vi "主界面.vi"() -> ()   [LabVIEW 2016]
uses:
  <vilib>/Utility/miscctls.llb/LVPointTypeDef.ctl
  <vilib>/NI/Modbus Library/API/Wrapper/Create Serial Slave.vi
  <vilib>/NI/Modbus Library/API/Slave/Modbus Slave.lvclass
  <vilib>/ptbypt/NI_PtbyPt.lvlib
  <vilib>/NI/Modbus Library/API/Wrapper/API Main.lvlib
panel:
  in  "质控单元串口重开":enum16{"不重开", "串口重开"}(ring)
  in  "采配水串口重开":enum16{"不重开", "串口重开"}(ring)
  out "质控运行中":bool
  out "质控单元通讯":bool
  out "采配水运行中":bool
  out "采配水通讯":bool
  out "CODCr运行中":bool
  out "CODMn运行中":bool
  out "总磷运行中":bool
  out "总氮运行中":bool
  out "氨氮运行中":bool
  out "CODCr通讯":bool
  out "CODMn通讯":bool
  out "总磷通讯":bool
  out "总氮通讯":bool
  out "氨氮通讯":bool
  out "系统日期/时间字符串":string
  in  "质控单元串口参数":T1={"VISA resource name"="COM28", "baud rate (设置)"=115200, "unit ID"=1}
  in  "采配水串口参数":T1={"VISA resource name"="COM23", "baud rate (设置)"=115200, "unit ID"=10}
  in  "质控单元":bool
  in  "采配水":bool
  in  "总磷串口参数":T1={"VISA resource name"="COM25", "baud rate (设置)"=115200, "unit ID"=1}
  in  "CODCr串口参数":T1={"VISA resource name"="COM29", "baud rate (设置)"=9600, "unit ID"=1}
  in  "CODMn串口参数":T1={"VISA resource name"="COM24", "baud rate (设置)"=115200, "unit ID"=1}
  in  "总氮串口参数":T1={"VISA resource name"="COM30", "baud rate (设置)"=115200, "unit ID"=2}
  in  "氨氮串口参数":T1={"VISA resource name"="COM27", "baud rate (设置)"=115200, "unit ID"=3}
  in  "CODCr":bool
  in  "CODMn":bool
  in  "总磷":bool
  in  "总氮":bool
  in  "氨氮":bool
  in  "CODCr串口重开":enum16{"不重开", "串口重开"}(ring)
  in  "CODMn串口重开":enum16{"不重开", "串口重开"}(ring)
  in  "总磷串口重开":enum16{"不重开", "串口重开"}(ring)
  in  "总氮串口重开":enum16{"不重开", "串口重开"}(ring)
  in  "氨氮串口重开":enum16{"不重开", "串口重开"}(ring)
  in  "退出":bool
  # "系统状态区"
  # "采配水"
  # "氨氮"
  # "总氮"
  # "总磷"
  # "CODMn"
  # "CODCr"
  # "质控单元"
  # "通讯状态："
  # "测量状态："
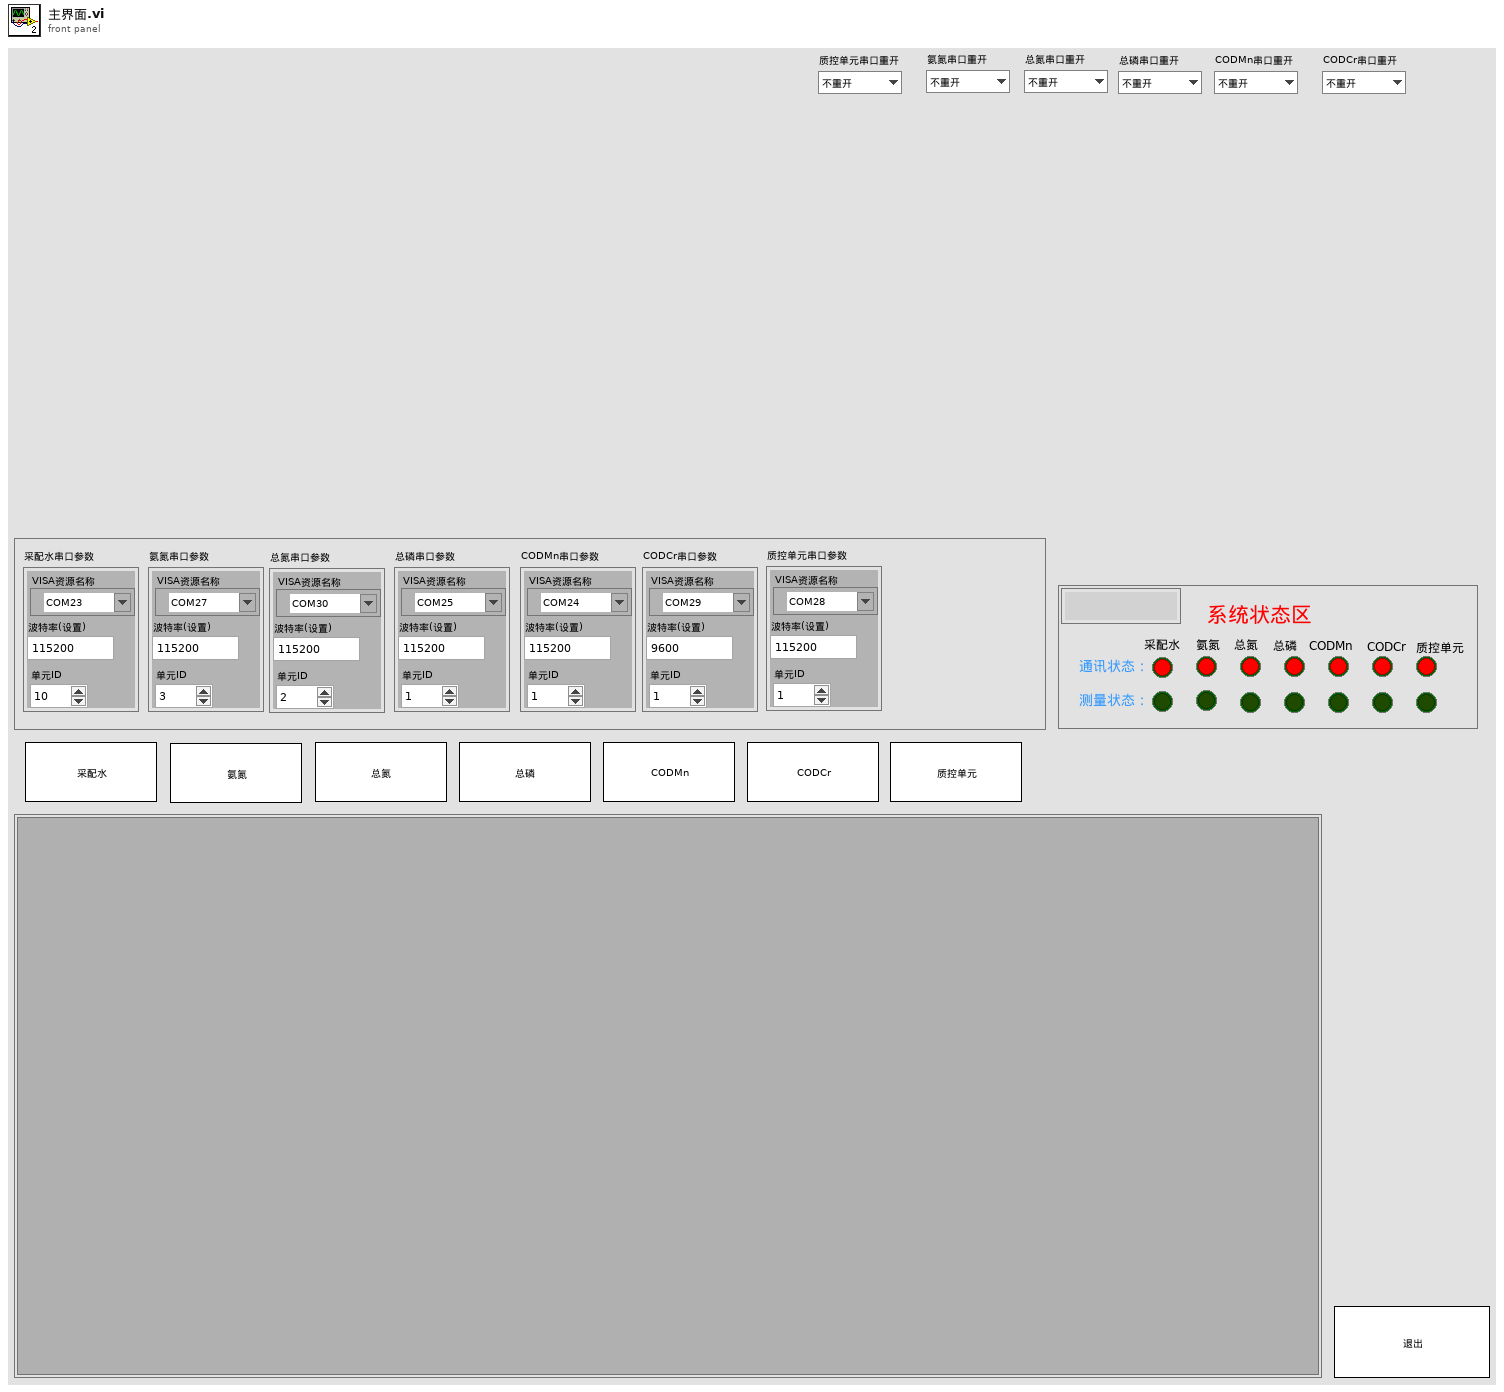
[diagram p1: front panel]
types:
  T1 = cluster{"VISA resource name":refnum<visa-resource-name>, "baud rate (设置)":u32, "unit ID":u8}
  T2 = enum16{"write register", "read register", "write and read register", "write coil", "read coil"}
  T3 = typedef "LVPointTypeDef.ctl" = cluster{"Horizontal":i16, "Vertical":i16}
  T4 = enum32{"Bad", "Idle", "Run top level", "Running"}
  T5 = cluster{"R0":i16, "R1":i16, "R2":i16, "R3":i16, "R4":i16}
  T6 = cluster{"因子编码":u32, "单位":u16, "标样参考值":sgl, "水样数据时间":timestamp, "水样实测值":sgl, "水样数据标识":string, "标样数据时间":timestamp, "标样实测值":sgl, "标样数据标识":string, "空白数据时间":timestamp, "空白实测值":sgl, "空白数据标识":string, "零点核查数据时间":timestamp, "零点核查实测值":sgl, "零点核查数据标识":string, "跨度核查数据时间":timestamp, "跨度核查实测值":sgl, "跨度核查数据标识":string, "加标回收数据时间":timestamp, "加标回收实测值":sgl, "加标回收数据标识":string, "平行样数据时间":timestamp, "平行样实测值":sgl, "平行样数据标识":string}
  T7 = cluster{"系统时间":timestamp, "工作状态":u16, "测量模式":u16, "告警代码":enum16{"无告警", "缺试剂告警", "缺水样告警", "缺蒸馏水告警", "缺标液告警", "仪表漏液告警", "标定异常告警", "超量程告警", "加热异常", "低试剂预警", "超上限告警", "超下限告警", "仪表内部其他异常", "滴定异常告警", "电极异常告警", "量程切换告警", "参数设置告警", "PH电极电位异常", "电导率电极异常", "浊度光度异常", "溶解氧电极异常", "溶解氧光强异常", "温度异常告警", "PH异常告警", "溶解氧异常告警", "电导率异常告警", "浊度异常告警", "叶绿素异常告警", "藻密度异常告警", "蓝绿藻异常告警", "ORP异常告警", "氨氮异常告警", "清洁刷异常告警", "SD卡异常告警", "蓝牙异常告警", "Wifi异常告警", "流程异常告警"}, "故障代码":enum16{"无故障", "电机故障", "温度故障", "通讯故障", "滴定故障"}, "日志代码":u16, "软件版本":u16, "F0":sgl, "F1":sgl, "F2":sgl, "F3":sgl, "T":sgl, "H":sgl, "id":u16, "flowid":u16, "量程":u16}
  T8 = enum16{"步骤1", "步骤2", "步骤3", "步骤4", "步骤5", "步骤6", "步骤7", "步骤8", "步骤9", "步骤10"}
  T9 = enum16{"步骤1", "步骤2", "步骤3", "步骤4", "步骤5", "步骤6", "步骤7", "步骤8", "步骤9", "步骤10"}[]
  T10 = cluster{"R100":i16, "R101":i16, "R102":i16, "R103":i16, "R104":i16, "R105":i16, "R106":i16, "R107":i16, "R108":i16, "R109":i16, "R110":i16, "R111":i16, "R112":i16, "R113":i16, "R114":i16, "R115":i16, "R116":i16, "R117":i16, "R118":i16, "R119":i16}
  T11 = cluster{"R0":i16, "R1":i16, "R2":i16, "R3":i16, "R4":i16, "R5":i16, "R6":i16, "R7":i16, "R8":i16, "R9":i16, "R10":i16, "R11":i16, "R12":i16, "R13":i16, "R14":i16, "R15":i16, "R16":i16, "R17":i16, "R18":i16, "R19":i16, "R20":i16, "R21":i16, "R22":i16, "R23":i16, "R24":i16, "R25":i16}
  T12 = cluster{"测量精度":u16, "消解温度":u16, "消解时长":u16, "量程下限":sgl, "量程上限":sgl, "曲线斜率K":sgl, "曲线斜率B":sgl, "标定日期":timestamp, "标液1浓度":sgl, "标液1测量过程值":sgl, "标液2浓度":sgl, "标液2测量过程值":sgl, "标液3浓度":sgl, "标液3测量过程值":sgl, "标液4浓度":sgl, "标液4测量过程值":sgl, "标液5浓度":sgl, "标液5测量过程值":sgl, "线性相关系数":sgl, "试剂余量":u32, "测量滴定值或吸光度":sgl, "空白校准时间":timestamp, "标样校准时间":timestamp, "检出限值":sgl, "校准系数":sgl, "设备系列号":string}
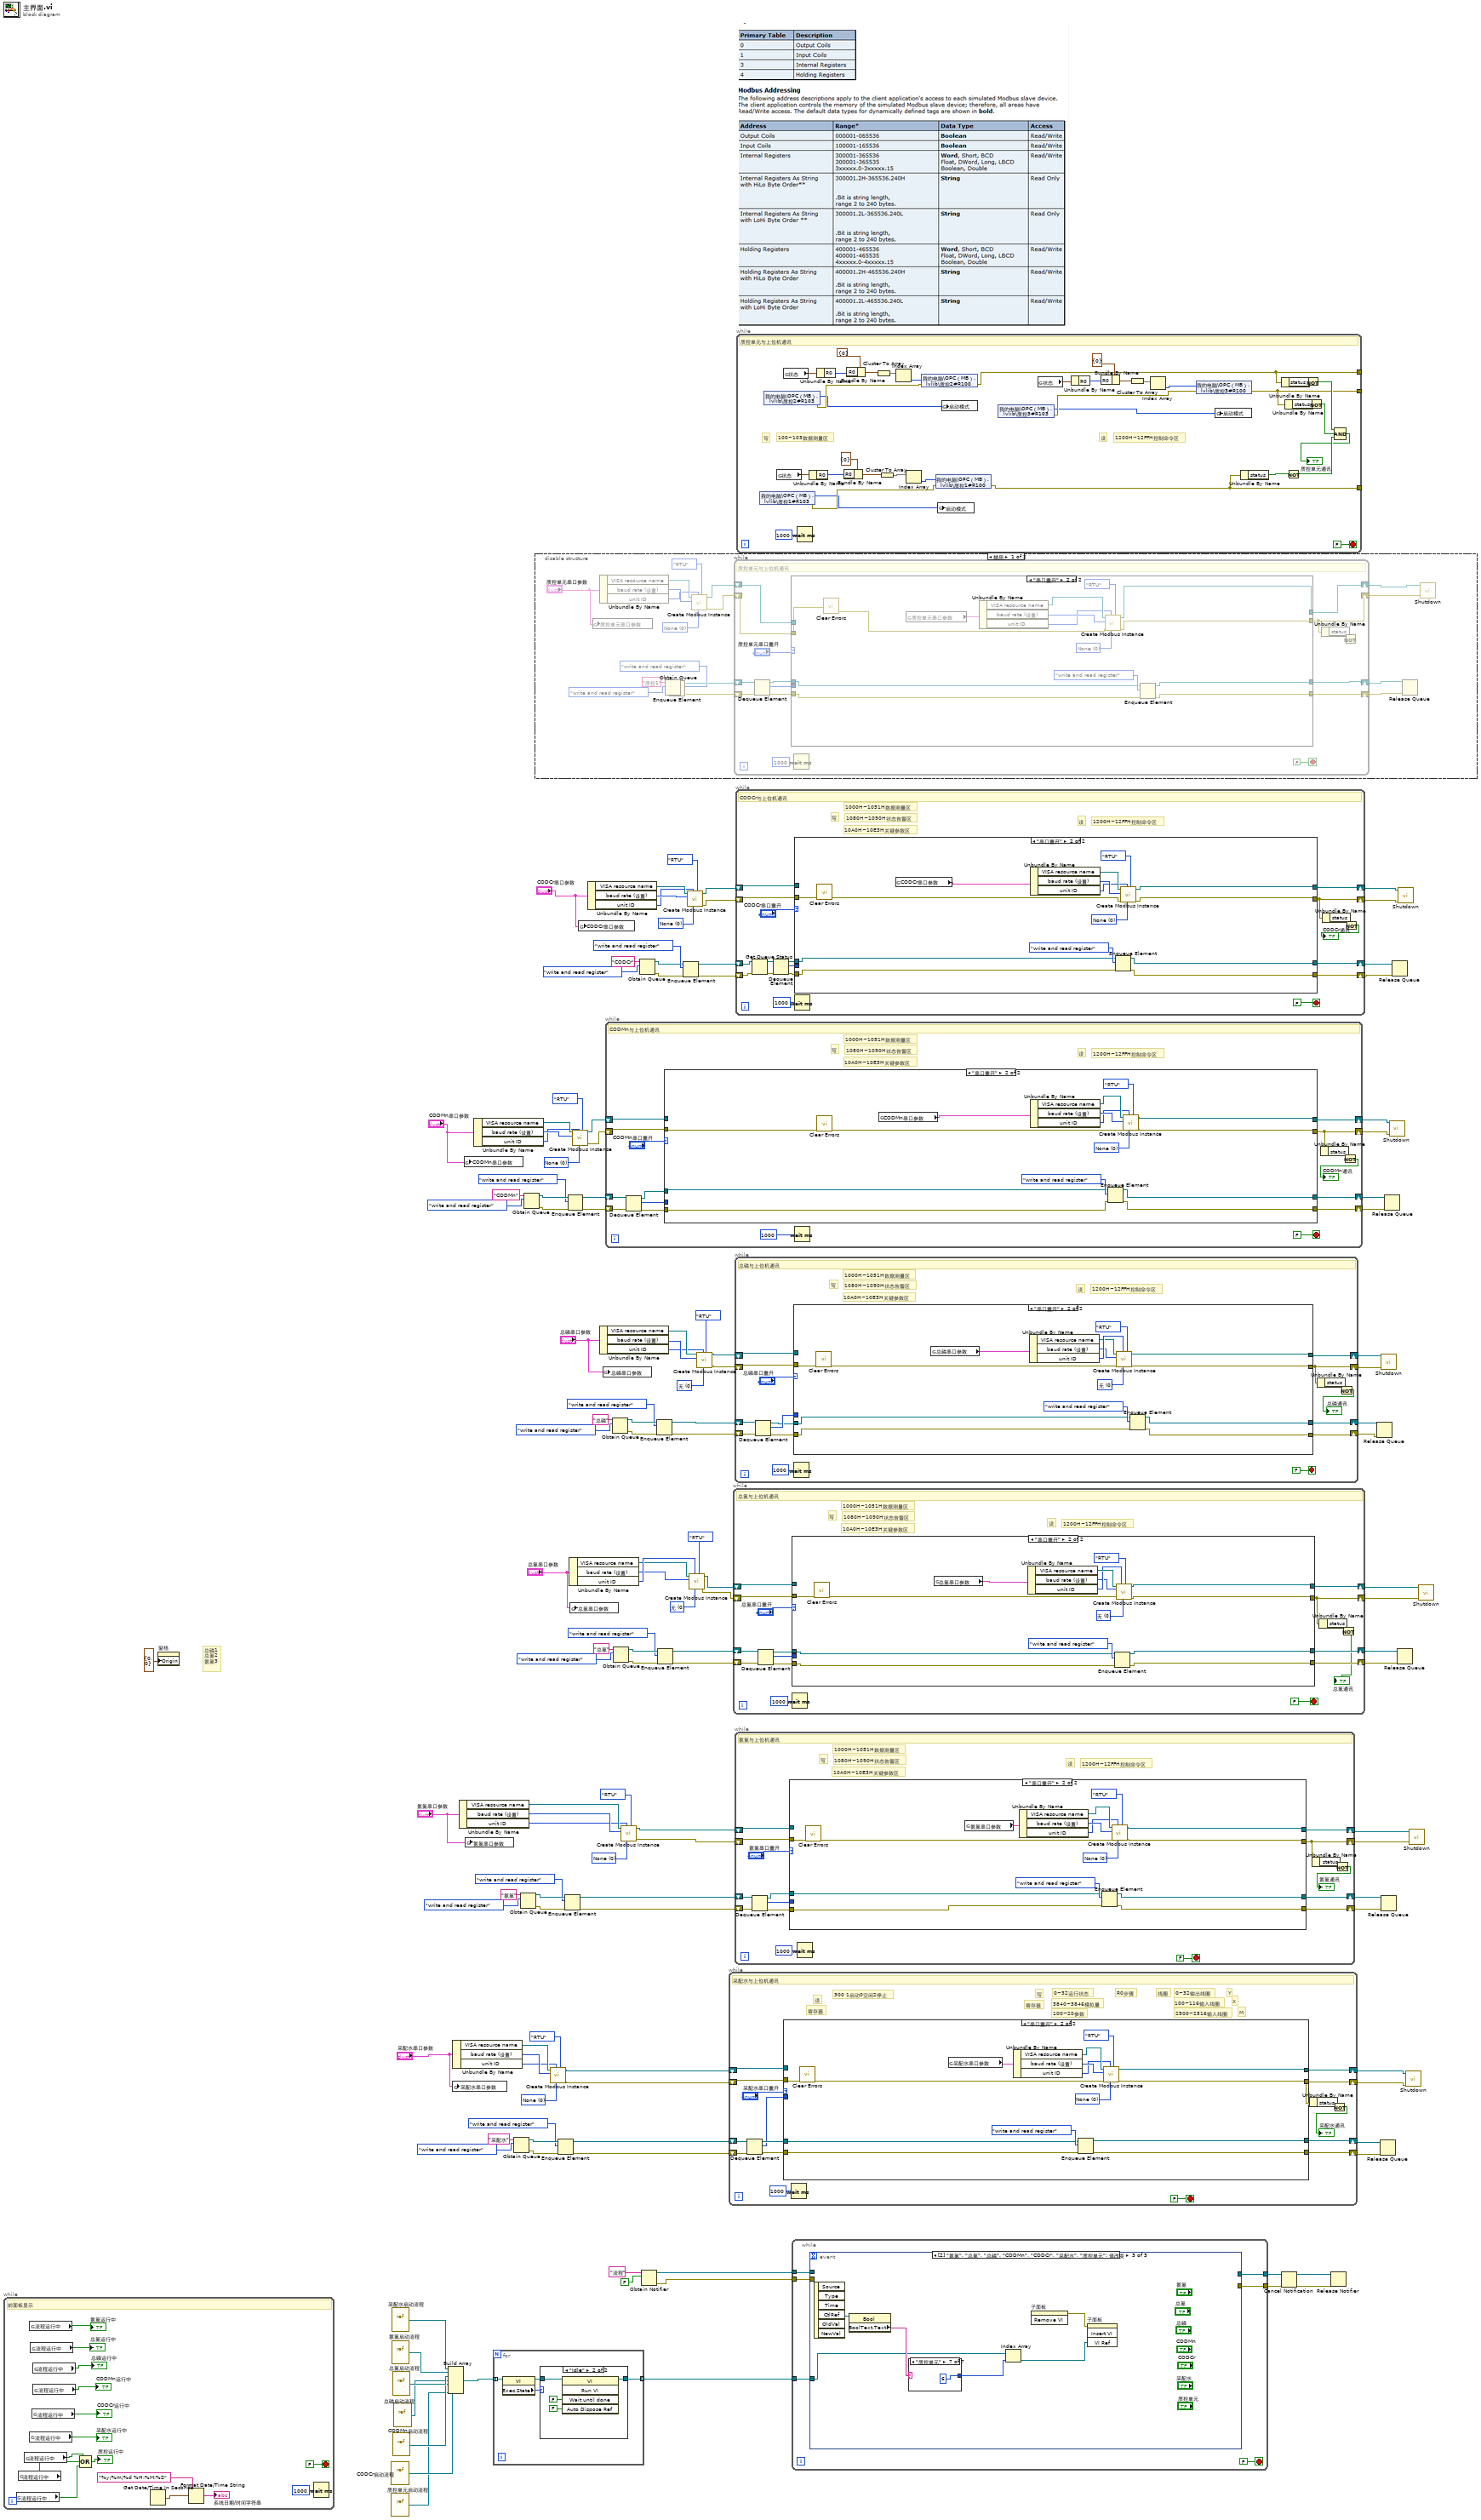
[diagram p0: block diagram]
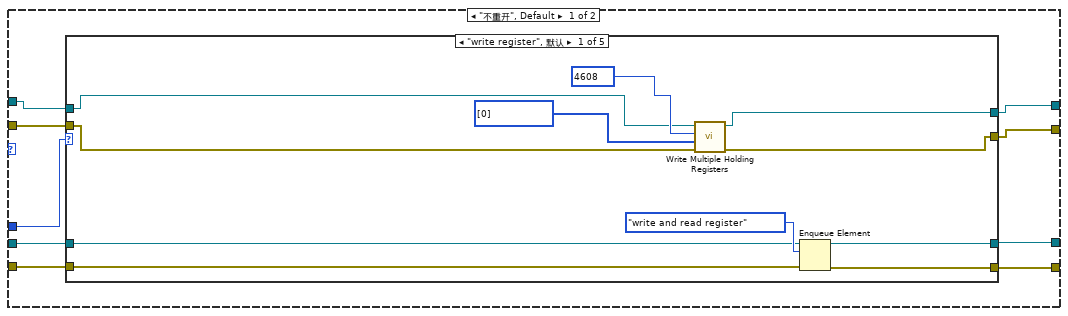
[diagram p2: hidden frame]
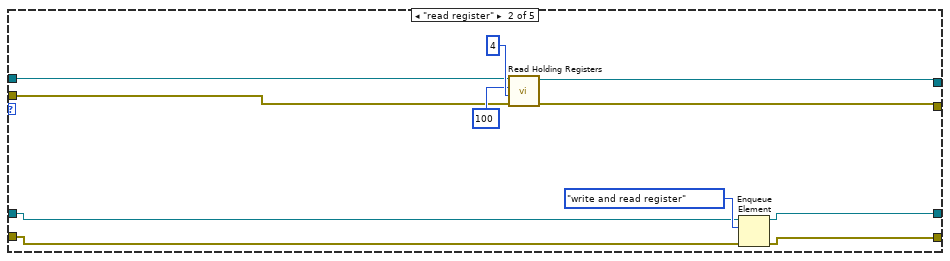
[diagram p3: hidden frame]
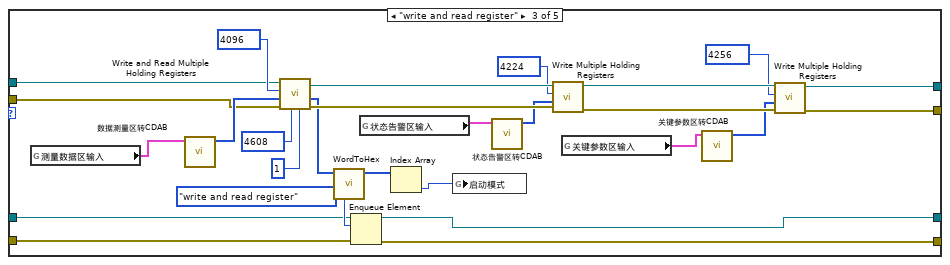
[diagram p4: hidden frame]
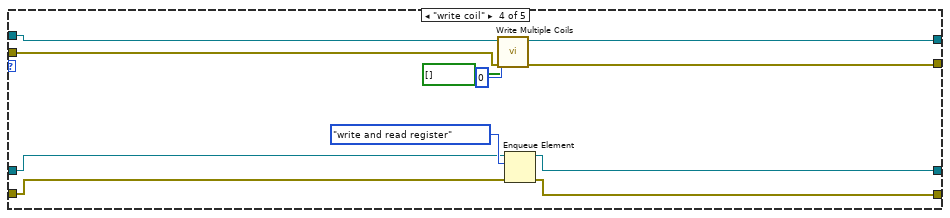
[diagram p5: hidden frame]
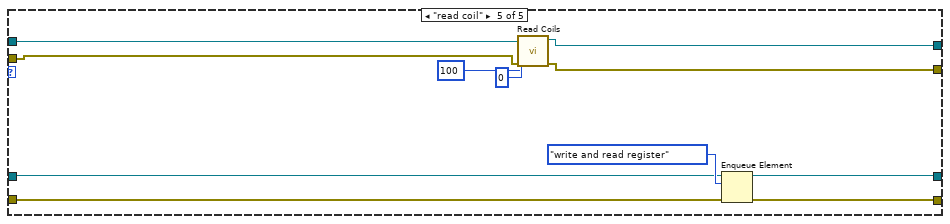
[diagram p6: hidden frame]
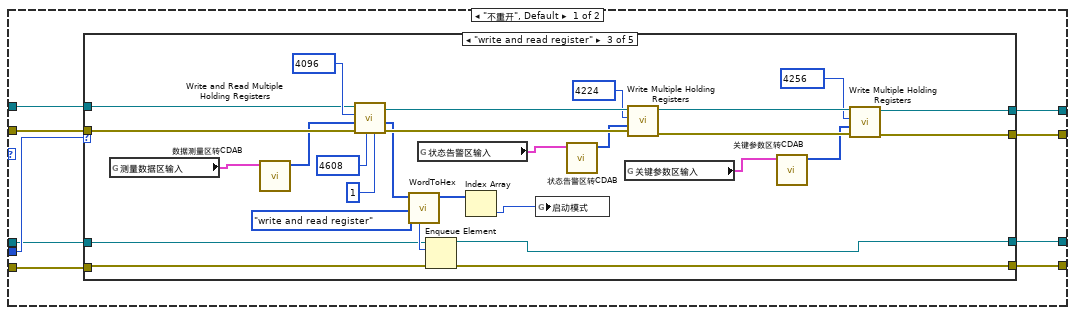
[diagram p7: hidden frame]
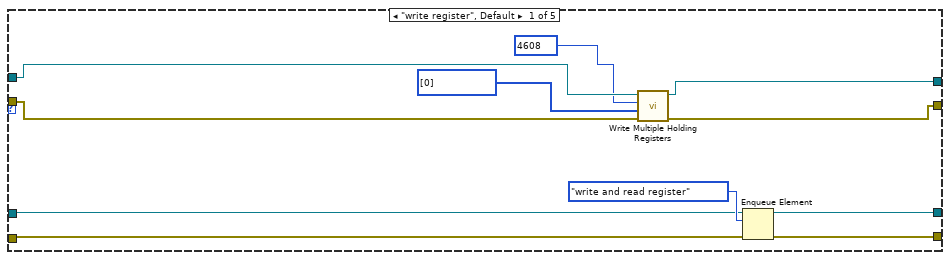
[diagram p8: hidden frame]
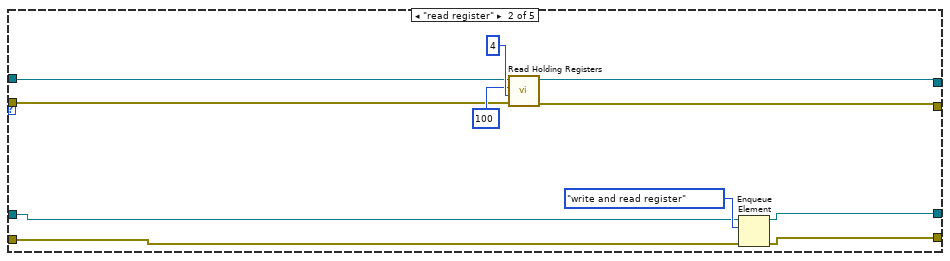
[diagram p9: hidden frame]
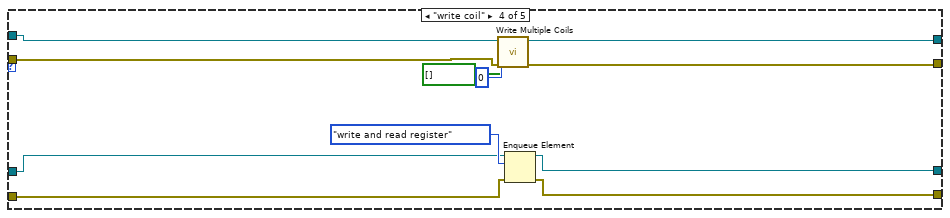
[diagram p10: hidden frame]
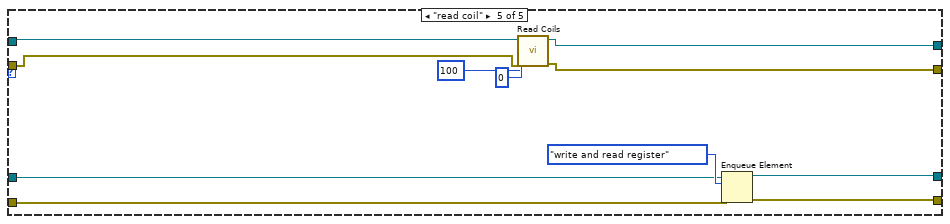
[diagram p11: hidden frame]
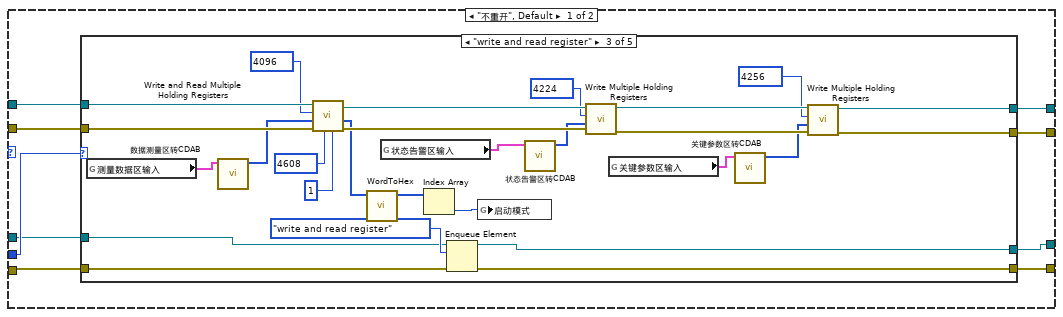
[diagram p12: hidden frame]
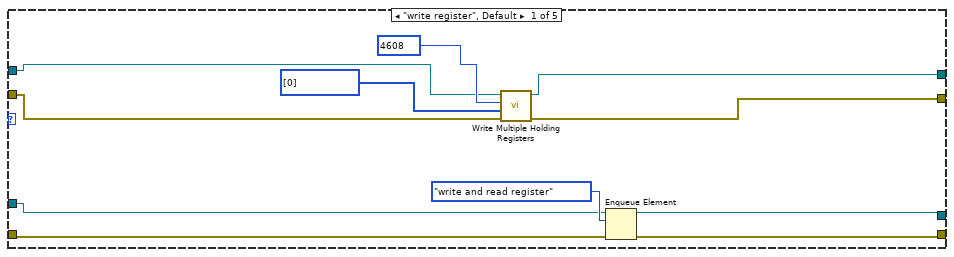
[diagram p13: hidden frame]
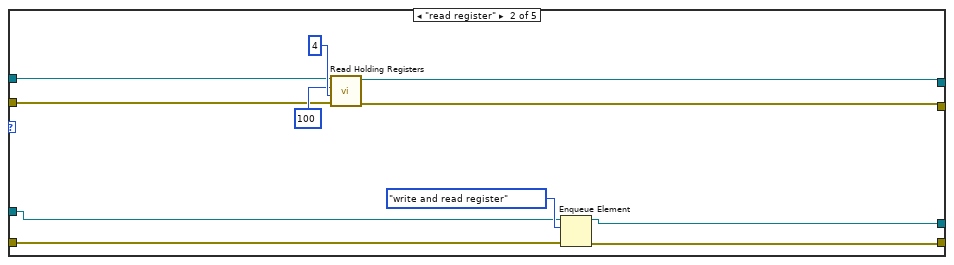
[diagram p14: hidden frame]
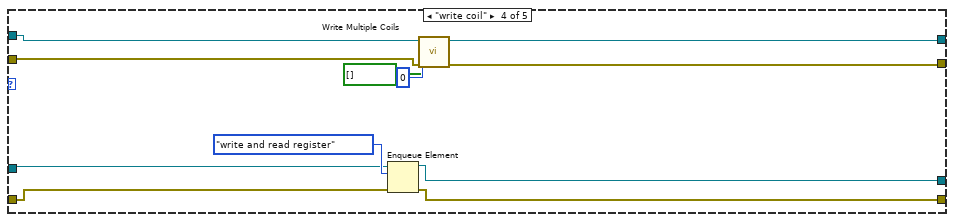
[diagram p15: hidden frame]
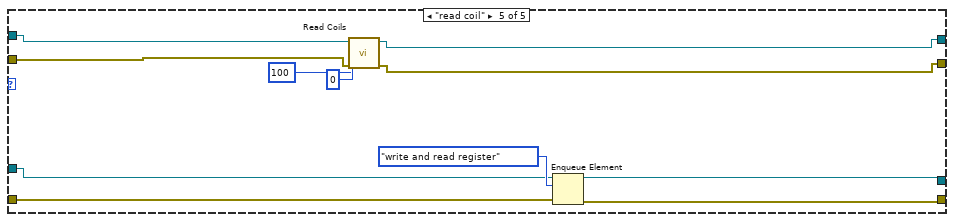
[diagram p16: hidden frame]
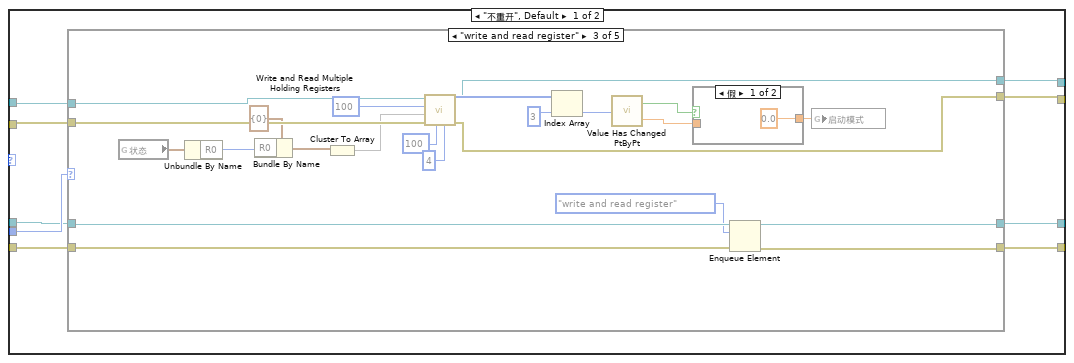
[diagram p17: hidden frame]
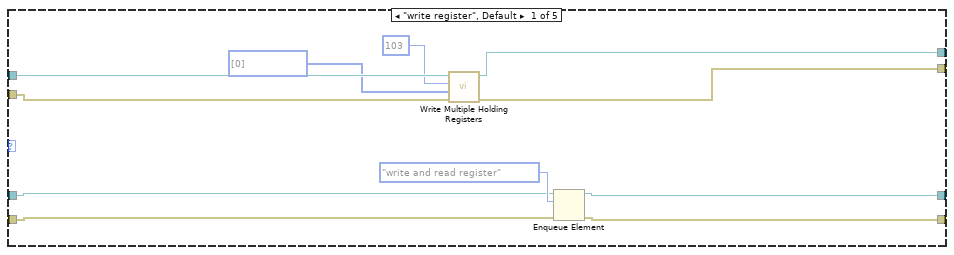
[diagram p18: hidden frame]
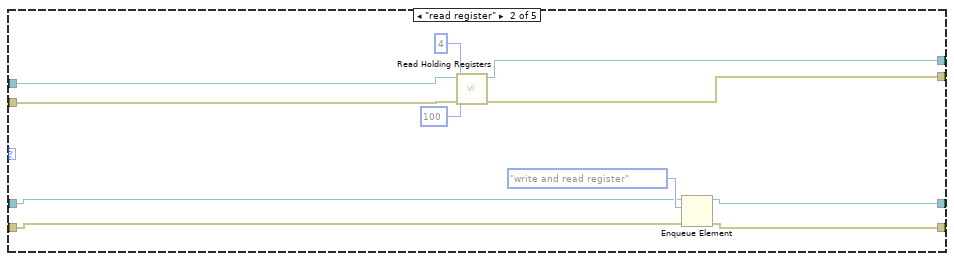
[diagram p19: hidden frame]
diagram:
  w6 = u16 0 items=["None", "Odd", "Even", "Mark", "Space"] ("parity (even)")
  w17 = u16 0 items=["None", "Odd", "Even", "Mark", "Space"] ("parity (even)")
  w26 = u16 0 items=["None", "Odd", "Even", "Mark", "Space"] ("parity (even)")
  w32 = u16 0 items=["None", "Odd", "Even", "Mark", "Space"] ("parity (even)")
  w39 = u16 0 items=["无", "奇", "偶"] ("parity (Even)")
  w44 = u16 0 items=["无", "奇", "偶"] ("parity (Even)")
  # "总磷1\n总氮2\n氨氮3"
  n1 = while {
    stop <- FALSE stop-if-true
    # "前面板显示"
    n2 = global read "质控单元3全局.vi" "流程运行中"() -> (w134:bool)
    n3 = global read "质控单元2全局.vi" "流程运行中"() -> (w135:bool)
    n4 = global read "质控单元全局.vi" "流程运行中"() -> (w136:bool)
    n5 = global read "氨氮全局.vi" "流程运行中"() -> (→"氨氮运行中":bool)
    n6 = global read "采配水全局.vi" "流程运行中"() -> (→"采配水运行中":bool)
    n7 = global read "总氮全局.vi" "流程运行中"() -> (→"总氮运行中":bool)
    n8 = global read "CODCr全局.vi" "流程运行中"() -> (→"CODCr运行中":bool)
    n9 = global read "总磷全局.vi" "流程运行中"() -> (→"总磷运行中":bool)
    n10 = global read "CODMn全局.vi" "流程运行中"() -> (→"CODMn运行中":bool)
    n11 = Compound Arithmetic op=OR ("复合运算")(w136, w135, w134) -> (→"质控运行中":bool)
    n12 = Get Date/Time In Seconds() -> (seconds since 1Jan1904=w143:timestamp)
    n13 = Format Date/Time String(time format string (%c)="%y/%m/%d %H:%M:%S" ("时间格式字符串(%c)"), seconds (now)=w143) -> (date/time string=→"系统日期/时间字符串":string)  [unwired: 1 in]
    n14 = Wait (ms)(milliseconds to wait=u32 1000 ("等待时间（毫秒）")) -> ()  [unwired: 1 out]
  }
  n15 = property on="窗格" class="Pane"("Origin"=T3 {"Horizontal"=0, "Vertical"=0} ("原点")) -> ()  [unwired: 2 in, 2 out]
  n16 = vi-ref "CODCr启动流程.vi"() -> (w115:refnum<vi>)
  n17 = vi-ref "质控单元启动流程.vi"() -> (w112:refnum<vi>)
  n18 = vi-ref "采配水启动流程.vi"() -> (w113:refnum<vi>)
  n19 = vi-ref "氨氮启动流程.vi"() -> (w119:refnum<vi>)
  n20 = vi-ref "总氮启动流程.vi"() -> (w118:refnum<vi>)
  n21 = vi-ref "CODMn启动流程.vi"() -> (w116:refnum<vi>)
  n22 = vi-ref "总磷启动流程.vi"() -> (w117:refnum<vi>)
  n23 = Build Array(w113, w119, w118, w117, w116, w115, w112) -> (w120:refnum<vi>[])
  n24 = global write "采配水全局.vi" "采配水串口参数"("采配水串口参数") -> ()
  n25 = Unbundle By Name("采配水串口参数") -> ("VISA resource name"=w25:refnum<visa-resource-name>, "baud rate (设置)"=w24:u32, "unit ID"=w23:u8)
  n26 = Unbundle By Name("氨氮串口参数") -> ("VISA resource name"=w36:refnum<visa-resource-name>, "baud rate (设置)"=w35:u32, "unit ID"=w34:u8)
  n27 = global write "CODMn全局.vi" "CODMn串口参数"("CODMn串口参数") -> ()
  n28 = global write "氨氮全局.vi" "氨氮串口参数"("氨氮串口参数") -> ()
  n29 = Unbundle By Name("CODMn串口参数") -> ("VISA resource name"=w16:refnum<visa-resource-name>, "baud rate (设置)"=w15:u32, "unit ID"=w14:u8)
  n30 = for {
    tunnel: [w149] -> w121 mode=indexing
    tunnel: w120 -> [w148] mode=indexing
    n31 = property class="VI"(reference=w148) -> (reference out=w150:refnum<vi>, "Exec.State"=w151:T4)  [unwired: 1 in, 1 out]
    n32 = case shown="\"Idle\"" w151 {
      tunnel: w150 -> [w152 w154]
      tunnel: [w152 w153] -> w149
      frame "Bad", Default {
      }
      frame "Idle" {
        n33 = invoke class="VI" method="Run VI"(reference=w154, "Wait until done"=FALSE ("结束前等待"), "Auto Dispose Ref"=FALSE ("自动销毁引用")) -> (reference out=w153:refnum<vi>)  [unwired: 2 in, 4 out]
      }
    }
  }
  n34 = Obtain Queue(name (unnamed)="采配水" ("名称（未命名）"), element data type=T2."write and read register") -> (queue out=w91:refnum<queue>, error out=w90:errorcluster)  [unwired: 3 in, 1 out]
  n35 = Obtain Queue(name (unnamed)="氨氮" ("名称（未命名）"), element data type=T2."write and read register") -> (queue out=w81:refnum<queue>, error out=w80:errorcluster)  [unwired: 3 in, 1 out]
  n36 = Obtain Queue(name (unnamed)="CODMn" ("名称（未命名）"), element data type=T2."write and read register") -> (queue out=w102:refnum<queue>, error out=w101:errorcluster)  [unwired: 3 in, 1 out]
  n37 = disable-structure shown="禁用" {
    frame Disabled {
      w164 = u16 0 items=["None", "Odd", "Even", "Mark", "Space"] ("parity (even)")
      n38 = global write "质控单元全局.vi" "质控单元串口参数"("质控单元串口参数") -> ()
      n39 = Unbundle By Name("质控单元串口参数") -> ("VISA resource name"=w161:refnum<visa-resource-name>, "baud rate (设置)"=w160:u32, "unit ID"=w159:u8)
      n40 = Obtain Queue(name (unnamed)="质控1" ("名称（未命名）"), element data type=T2."write and read register") -> (queue out=w172:refnum<queue>, error out=w171:errorcluster)  [unwired: 3 in, 1 out]
      n41 = Enqueue Element(queue=w172, element=T2."write and read register", error in (no error)=w171) -> (queue out=w169:refnum<queue>, error out=w168:errorcluster)  [unwired: 1 in, 1 out]
      n42 = call-poly <vilib>:"Create Modbus Instance.vi"("serial type"=enum16{"RTU", "ASCII"}."RTU", "parity (even)"=w164, "unit ID"=w159, "baud rate (9600)"=w160, "VISA resource name"=w161) -> ("error out"=w162:errorcluster, "serial slave instance"=w163:refnum<class "Modbus Slave.lvclass">)  [unwired: 5 in]
      n43 = while "While循环" {
        shift-right: [w187] -> w158
        shift-left: w163 -> [w190]
        shift-right: [w183] -> w157
        shift-left: w162 -> [w189]
        shift-right: [w177] -> w167
        shift-left: w169 -> [w181]
        shift-right: [w176] -> w166
        shift-left: w168 -> [w182]
        stop <- FALSE stop-if-true
        # "质控单元与上位机通讯"
        n44 = Dequeue Element(queue=w181, error in (no error)=w182) -> (queue out=w179:refnum<queue>, element=w180:T2, error out=w178:errorcluster)  [unwired: 1 in, 1 out]
        n45 = case shown="\"串口重开\"" "质控单元串口重开" {
          tunnel: w190 -> [w198 _]
          tunnel: w189 -> [w199 w283]
          tunnel: [w197 w270] -> w187
          tunnel: [w196 w271] -> w183
          tunnel: w180 -> [w195 _]
          tunnel: w179 -> [w194 w280]
          tunnel: w178 -> [w193 w279]
          tunnel: [w192 w278] -> w177
          tunnel: [w191 w277] -> w176
          frame "不重开", Default {
            n46 = case shown="\"write and read register\"" w195 {
              tunnel: w199 -> [w204 w215 w244 w251 w262]
              tunnel: w198 -> [w205 w216 w239 w252 w263]
              tunnel: [w201 w214 w232 w250 w261] -> w197
              tunnel: [w200 w213 w231 w249 w260] -> w196
              tunnel: w194 -> [w209 w220 w226 w256 w267]
              tunnel: w193 -> [w208 w219 w225 w255 w266]
              tunnel: [w207 w218 w224 w254 w265] -> w192
              tunnel: [w206 w217 w223 w253 w264] -> w191
              frame "write register", Default {
                n47 = call-dynamic "Write Multiple Holding Registers.vi"("error in"=w204, "registers to write"=u16[] [0] ("holding register values"), "starting address"=u16 103, "Modbus slave in"=w205) -> ("error out"=w200:errorcluster, "Modbus slave out"=w201:refnum<class "Modbus Slave.lvclass">)  [unwired: 6 in]
                n48 = Enqueue Element(queue=w209, element=T2."write and read register", error in (no error)=w208) -> (queue out=w207:refnum<queue>, error out=w206:errorcluster)  [unwired: 1 in, 1 out]
              }
              frame "read register" {
                n49 = call-dynamic "Read Holding Registers.vi"("error in"=w215, "number of inputs"=u16 4 ("number of holding registers"), "starting address"=u16 100, "Modbus slave in"=w216) -> ("error out"=w213:errorcluster, "Modbus slave out"=w214:refnum<class "Modbus Slave.lvclass">)  [unwired: 5 in, 1 out]
                n50 = Enqueue Element(queue=w220, element=T2."write and read register", error in (no error)=w219) -> (queue out=w218:refnum<queue>, error out=w217:errorcluster)  [unwired: 1 in, 1 out]
              }
              frame "write and read register" {
                n51 = global read "质控单元全局.vi" "状态"() -> (w228:T5)
                n52 = Unbundle By Name(w228) -> ("R0"=w227:i16)
                n53 = Bundle By Name(cluster=cluster{"R0":i16} {"R0"=0} ("状态"), "R0"=w227) -> (w229:cluster{"R0":i16})
                n54 = Cluster To Array(cluster=w229) -> (array=w236:i16[])
                n55 = call-dynamic "Write and Read Multiple Holding Registers.vi"("read count"=u16 4, "read starting address"=u16 100 ("read count"), "error in"=w244, "write values"=w236, "write starting address"=u16 100 ("read count"), "Modbus instance in"=w239) -> ("error out"=w231:errorcluster, "read values"=w237:u16[], "Modbus instance out"=w232:refnum<class "Modbus Slave.lvclass">)  [unwired: 3 in]
                n56 = Index Array(array=w237, index=3 ("索引")) -> (element=w242:u16)
                n57 = call <vilib>:"Value Has Changed PtByPt.vi"("input data point"=w242) -> ("has changed"=w241:bool, "output data point"=w240:dbl)  [unwired: 1 in]
                n58 = case shown="假" w241 {
                  tunnel: [0.0 ("output data point") w246] -> w233
                  tunnel: w240 -> [_ w246]
                  frame False {
                  }
                  frame True {
                  }
                }
                n59 = Enqueue Element(queue=w226, element=T2."write and read register", error in (no error)=w225) -> (queue out=w224:refnum<queue>, error out=w223:errorcluster)  [unwired: 1 in, 1 out]
                n60 = global write "质控单元全局.vi" "启动模式"(w233) -> ()
              }
              frame "write coil" {
                n61 = call-dynamic "Write Multiple Coils.vi"("error in"=w251, "coils to write"=bool[] [] ("coil values"), "starting address"=u16 0, "Modbus slave in"=w252) -> ("error out"=w249:errorcluster, "Modbus slave out"=w250:refnum<class "Modbus Slave.lvclass">)  [unwired: 6 in]
                n62 = Enqueue Element(queue=w256, element=T2."write and read register", error in (no error)=w255) -> (queue out=w254:refnum<queue>, error out=w253:errorcluster)  [unwired: 1 in, 1 out]
              }
              frame "read coil" {
                n63 = call-dynamic "Read Coils.vi"("error in"=w262, "number of inputs"=u16 100 ("number of coils"), "starting address"=u16 0, "Modbus slave in"=w263) -> ("error out"=w260:errorcluster, "Modbus slave out"=w261:refnum<class "Modbus Slave.lvclass">)  [unwired: 5 in, 1 out]
                n64 = Enqueue Element(queue=w267, element=T2."write and read register", error in (no error)=w266) -> (queue out=w265:refnum<queue>, error out=w264:errorcluster)  [unwired: 1 in, 1 out]
              }
            }
          }
          frame "串口重开" {
            w275 = u16 0 items=["None", "Odd", "Even", "Mark", "Space"] ("parity (even)")
            n65 = call <vilib>:"Clear Errors.vi"("error in (no error)"=w283) -> ("error out"=w272:errorcluster)  [unwired: 5 in, 1 out]
            n66 = global read "质控单元全局.vi" "质控单元串口参数"() -> (w282:T1)
            n67 = Unbundle By Name(w282) -> ("VISA resource name"=w274:refnum<visa-resource-name>, "baud rate (设置)"=w273:u32, "unit ID"=w269:u8)
            n68 = call-poly <vilib>:"Create Modbus Instance.vi"("serial type"=enum16{"RTU", "ASCII"}."RTU", "parity (even)"=w275, "unit ID"=w269, "error in"=w272, "baud rate (9600)"=w273, "VISA resource name"=w274) -> ("error out"=w271:errorcluster, "serial slave instance"=w270:refnum<class "Modbus Slave.lvclass">)  [unwired: 4 in]
            n69 = Enqueue Element(queue=w280, element=T2."write and read register", error in (no error)=w279) -> (queue out=w278:refnum<queue>, error out=w277:errorcluster)  [unwired: 1 in, 1 out]
          }
        }
        n70 = Wait (ms)(milliseconds to wait=u32 1000 ("等待时间（毫秒）")) -> ()  [unwired: 1 out]
        n71 = Unbundle By Name(w183) -> ("status"=w184:bool)
        n72 = Not(x=w184) -> ()  [unwired: 1 out]
      }
      n73 = Release Queue(queue=w167, error in (no error)=w166) -> ()  [unwired: 1 in, 3 out]
      n74 = call-dynamic "Shutdown.vi"("error in"=w157, "Modbus slave in"=w158) -> ()  [unwired: 9 in, 1 out]
    }
    frame Enabled {
    }
  }
  n75 = call-poly <vilib>:"Create Modbus Instance.vi"("serial type"=enum16{"RTU", "ASCII"}."RTU", "parity (even)"=w26, "unit ID"=w23, "baud rate (9600)"=w24, "VISA resource name"=w25) -> ("error out"=w21:errorcluster, "serial slave instance"=w22:refnum<class "Modbus Slave.lvclass">)  [unwired: 5 in]
  n76 = Enqueue Element(queue=w91, element=T2."write and read register", error in (no error)=w90) -> (queue out=w88:refnum<queue>, error out=w87:errorcluster)  [unwired: 1 in, 1 out]
  n77 = Enqueue Element(queue=w81, element=T2."write and read register", error in (no error)=w80) -> (queue out=w78:refnum<queue>, error out=w77:errorcluster)  [unwired: 1 in, 1 out]
  n78 = Enqueue Element(queue=w102, element=T2."write and read register", error in (no error)=w101) -> (queue out=w99:refnum<queue>, error out=w98:errorcluster)  [unwired: 1 in, 1 out]
  n79 = Unbundle By Name("总氮串口参数") -> ("VISA resource name"=w41:refnum<visa-resource-name>, "baud rate (设置)"=w40:u32, "unit ID"=w53:u8)
  n80 = global write "总氮全局.vi" "总氮串口参数"("总氮串口参数") -> ()
  n81 = call-poly <vilib>:"Create Modbus Instance.vi"("serial type"=enum16{"RTU", "ASCII"}."RTU", "parity (even)"=w17, "unit ID"=w14, "baud rate (9600)"=w15, "VISA resource name"=w16) -> ("error out"=w12:errorcluster, "serial slave instance"=w13:refnum<class "Modbus Slave.lvclass">)  [unwired: 5 in]
  n82 = global write "CODCr全局.vi" "CODCr串口参数"("CODCr串口参数") -> ()
  n83 = Unbundle By Name("CODCr串口参数") -> ("VISA resource name"=w5:refnum<visa-resource-name>, "baud rate (设置)"=w4:u32, "unit ID"=w3:u8)
  n84 = Unbundle By Name("总磷串口参数") -> ("VISA resource name"=w49:refnum<visa-resource-name>, "baud rate (设置)"=w48:u32, "unit ID"=w47:u8)
  n85 = global write "总磷全局.vi" "总磷串口参数"("总磷串口参数") -> ()
  n86 = while "While循环" {
    shift-right: [w297] -> w11
    shift-left: w13 -> [w284]
    shift-right: [w292] -> w10
    shift-left: w12 -> [w299]
    shift-right: [w286] -> w95
    shift-left: w99 -> [w291]
    shift-right: [w285] -> w94
    shift-left: w98 -> [w290]
    stop <- FALSE stop-if-true
    # "1200H~12FFH控制命令区"
    # "读"
    # "写"
    # "10A0H~10E3H关键参数区"
    # "1080H~1090H状态告警区"
    # "1000H~1051H数据测量区"
    # "CODMn与上位机通讯"
    n87 = Dequeue Element(queue=w291, error in (no error)=w290) -> (queue out=w288:refnum<queue>, element=w289:T2, error out=w287:errorcluster)  [unwired: 1 in, 1 out]
    n88 = case shown="\"串口重开\"" "CODMn串口重开" {
      tunnel: w299 -> [w308 w421]
      tunnel: [w307 w407] -> w297
      tunnel: [w306 w408] -> w292
      tunnel: w289 -> [w305 _]
      tunnel: w288 -> [w304 w418]
      tunnel: w287 -> [w303 w417]
      tunnel: [w302 w416] -> w286
      tunnel: [w301 w415] -> w285
      tunnel: w284 -> [w300 _]
      frame "不重开", Default {
        n89 = case shown="\"write and read register\"" w305 {
          tunnel: w308 -> [w317 w324 w366 w392 w403]
          tunnel: [w316 w321 w357 w391 w402] -> w307
          tunnel: [w315 w320 w356 w390 w401] -> w306
          tunnel: w304 -> [w314 w329 w352 w389 w400]
          tunnel: w303 -> [w313 w328 w351 w388 w399]
          tunnel: [w312 w327 w350 w387 w398] -> w302
          tunnel: [w311 w326 w349 w386 w397] -> w301
          tunnel: w300 -> [w309 w323 w348 w385 w396]
          frame "write register", Default {
            n90 = call-dynamic "Write Multiple Holding Registers.vi"("error in"=w317, "registers to write"=u16[] [0] ("holding register values"), "starting address"=u16 4608 ("write operation starting address"), "Modbus slave in"=w309) -> ("error out"=w315:errorcluster, "Modbus slave out"=w316:refnum<class "Modbus Slave.lvclass">)  [unwired: 6 in]
            n91 = Enqueue Element(queue=w314, element=T2."write and read register", error in (no error)=w313) -> (queue out=w312:refnum<queue>, error out=w311:errorcluster)  [unwired: 1 in, 1 out]
          }
          frame "read register" {
            n92 = call-dynamic "Read Holding Registers.vi"("error in"=w324, "number of inputs"=u16 4 ("number of holding registers"), "starting address"=u16 100, "Modbus slave in"=w323) -> ("error out"=w320:errorcluster, "Modbus slave out"=w321:refnum<class "Modbus Slave.lvclass">)  [unwired: 5 in, 1 out]
            n93 = Enqueue Element(queue=w329, element=T2."write and read register", error in (no error)=w328) -> (queue out=w327:refnum<queue>, error out=w326:errorcluster)  [unwired: 1 in, 1 out]
          }
          frame "write and read register" {
            n94 = global read "CODMn全局.vi" "启动命令（模式）"() -> (w333:string)
            n95 = global read "CODMn全局.vi" "测量数据区输入"() -> (w334:T6)
            n96 = case shown="\"加标回收\"" w333 {
              tunnel: w334 -> [w368 w370 w372 w374 w376 w378 w380 w382 w384]
              tunnel: [w367 w369 w371 w373 w375 w377 w379 w381 w383] -> w332
              frame "水样测量", Default {
                n97 = Unbundle By Name(w368) -> ("水样实测值"=w367:sgl)
              }
              frame "标样核查" {
                n98 = Unbundle By Name(w370) -> ("标样实测值"=w369:sgl)
              }
              frame "零点核查" {
                n99 = Unbundle By Name(w372) -> ("空白实测值"=w371:sgl)
              }
              frame "跨度核查" {
                n100 = Unbundle By Name(w374) -> ("跨度核查实测值"=w373:sgl)
              }
              frame "空白测试" {
                n101 = Unbundle By Name(w376) -> ("空白实测值"=w375:sgl)
              }
              frame "平行样测试" {
                n102 = Unbundle By Name(w378) -> ("平行样实测值"=w377:sgl)
              }
              frame "加标回收" {
                n103 = Unbundle By Name(w380) -> ("加标回收实测值"=w379:sgl)
              }
              frame "空白校准" {
                n104 = Unbundle By Name(w382) -> ("空白实测值"=w381:sgl)
              }
              frame "标样校准" {
                n105 = Unbundle By Name(w384) -> ("标样实测值"=w383:sgl)
              }
            }
            n106 = Multiply(x=w332, y=sgl 100.0) -> (x*y=w342:sgl)
            n107 = To Long Integer(number=w342) -> (32bit integer=w343:i32)
            n108 = Build Array(w343) -> (w339:i32[])
            n109 = call-dynamic "Write and Read Multiple Holding Registers.vi"("read count"=u16 1, "read starting address"=u16 4608 ("write operation starting address"), "error in"=w366, "write values"=w339, "write starting address"=u16 4104 ("write operation starting address"), "Modbus instance in"=w348) -> ("error out"=w361:errorcluster, "read values"=w354:u16[], "Modbus instance out"=w362:refnum<class "Modbus Slave.lvclass">)  [unwired: 3 in]
            n110 = global read "CODMn全局.vi" "状态告警区输入"() -> (w347:T7)
            n111 = Index Array(array=w354) -> (element=w331:u16)  [unwired: 1 in]
            n112 = Unbundle By Name(w347) -> ("系统时间"=w338:timestamp, "工作状态"=w346:u16)
            n113 = Enqueue Element(queue=w352, element=T2."write and read register", error in (no error)=w351) -> (queue out=w350:refnum<queue>, error out=w349:errorcluster)  [unwired: 1 in, 1 out]
            n114 = Build Array(w338) -> (w337:timestamp[])
            n115 = Build Array(w346) -> (w336:u16[])
            n116 = call "DateToHex.vi"("DATE"=w337) -> ("数组"=w340:u16[])  [unwired: 10 in]
            n117 = global write "CODMn全局.vi" "启动模式"(w331) -> ()
            n118 = Insert Into Array(array=w340, new element=w336) -> (w335:u16[])  [unwired: 1 in]
            n119 = call-dynamic "Write Multiple Holding Registers.vi"("error in"=w361, "registers to write"=w335, "starting address"=u16 4224 ("write operation starting address"), "Modbus slave in"=w362) -> ("error out"=w358:errorcluster, "Modbus slave out"=w359:refnum<class "Modbus Slave.lvclass">)  [unwired: 6 in]
            n120 = global read "CODMn全局.vi" "当前步骤"() -> (w345:T8)
            n121 = Build Array(w345) -> (w344:T9)
            n122 = call-dynamic "Write Multiple Holding Registers.vi"("error in"=w358, "registers to write"=w344, "starting address"=u16 4239 ("write operation starting address"), "Modbus slave in"=w359) -> ("error out"=w356:errorcluster, "Modbus slave out"=w357:refnum<class "Modbus Slave.lvclass">)  [unwired: 6 in]
          }
          frame "write coil" {
            n123 = call-dynamic "Write Multiple Coils.vi"("error in"=w392, "coils to write"=bool[] [] ("coil values"), "starting address"=u16 0, "Modbus slave in"=w385) -> ("error out"=w390:errorcluster, "Modbus slave out"=w391:refnum<class "Modbus Slave.lvclass">)  [unwired: 6 in]
            n124 = Enqueue Element(queue=w389, element=T2."write and read register", error in (no error)=w388) -> (queue out=w387:refnum<queue>, error out=w386:errorcluster)  [unwired: 1 in, 1 out]
          }
          frame "read coil" {
            n125 = call-dynamic "Read Coils.vi"("error in"=w403, "number of inputs"=u16 100 ("number of coils"), "starting address"=u16 0, "Modbus slave in"=w396) -> ("error out"=w401:errorcluster, "Modbus slave out"=w402:refnum<class "Modbus Slave.lvclass">)  [unwired: 5 in, 1 out]
            n126 = Enqueue Element(queue=w400, element=T2."write and read register", error in (no error)=w399) -> (queue out=w398:refnum<queue>, error out=w397:errorcluster)  [unwired: 1 in, 1 out]
          }
        }
      }
      frame "串口重开" {
        w413 = u16 0 items=["None", "Odd", "Even", "Mark", "Space"] ("parity (even)")
        n127 = call <vilib>:"Clear Errors.vi"("error in (no error)"=w421) -> ("error out"=w409:errorcluster)  [unwired: 5 in, 1 out]
        n128 = global read "CODMn全局.vi" "CODMn串口参数"() -> (w420:T1)
        n129 = Unbundle By Name(w420) -> ("VISA resource name"=w412:refnum<visa-resource-name>, "baud rate (设置)"=w411:u32, "unit ID"=w410:u8)
        n130 = Enqueue Element(queue=w418, element=T2."write and read register", error in (no error)=w417) -> (queue out=w416:refnum<queue>, error out=w415:errorcluster)  [unwired: 1 in, 1 out]
        n131 = call-poly <vilib>:"Create Modbus Instance.vi"("serial type"=enum16{"RTU", "ASCII"}."RTU", "parity (even)"=w413, "unit ID"=w410, "error in"=w409, "baud rate (9600)"=w411, "VISA resource name"=w412) -> ("error out"=w408:errorcluster, "serial slave instance"=w407:refnum<class "Modbus Slave.lvclass">)  [unwired: 4 in]
      }
    }
    n132 = Wait (ms)(milliseconds to wait=u32 1000 ("等待时间（毫秒）")) -> ()  [unwired: 1 out]
    n133 = Unbundle By Name(w292) -> ("status"=w294:bool)
    n134 = Not(x=w294) -> (.not. x?=→"CODMn通讯":bool)
  }
  n135 = Obtain Queue(name (unnamed)="总磷" ("名称（未命名）"), element data type=T2."write and read register") -> (queue out=w61:refnum<queue>, error out=w60:errorcluster)  [unwired: 3 in, 1 out]
  n136 = Obtain Queue(name (unnamed)="总氮" ("名称（未命名）"), element data type=T2."write and read register") -> (queue out=w71:refnum<queue>, error out=w70:errorcluster)  [unwired: 3 in, 1 out]
  n137 = call-poly <vilib>:"Create Modbus Instance.vi"("serial type"=enum16{"RTU", "ASCII"}."RTU", "parity (even)"=w32, "unit ID"=w34, "baud rate (9600)"=w35, "VISA resource name"=w36) -> ("error out"=w30:errorcluster, "serial slave instance"=w31:refnum<class "Modbus Slave.lvclass">)  [unwired: 5 in]
  n138 = Obtain Queue(name (unnamed)="CODCr" ("名称（未命名）"), element data type=T2."write and read register") -> (queue out=w109:refnum<queue>, error out=w110:errorcluster)  [unwired: 3 in, 1 out]
  n139 = Obtain Notifier(name (unnamed)="流程" ("名称（未命名）"), notification data type=FALSE) -> (notifier out=w128:refnum<notifier>, error out=w127:errorcluster)  [unwired: 2 in, 1 out]
  n140 = Enqueue Element(queue=w61, element=T2."write and read register", error in (no error)=w60) -> (queue out=w58:refnum<queue>, error out=w57:errorcluster)  [unwired: 1 in, 1 out]
  n141 = Enqueue Element(queue=w71, element=T2."write and read register", error in (no error)=w70) -> (queue out=w68:refnum<queue>, error out=w67:errorcluster)  [unwired: 1 in, 1 out]
  n142 = Enqueue Element(queue=w109, element=T2."write and read register", error in (no error)=w110) -> (queue out=w106:refnum<queue>, error out=w105:errorcluster)  [unwired: 1 in, 1 out]
  n143 = call-poly <vilib>:"Create Modbus Instance.vi"("serial type"=enum16{"RTU", "ASCII"}."RTU", "parity (even)"=w6, "unit ID"=w3, "baud rate (9600)"=w4, "VISA resource name"=w5) -> ("error out"=w1:errorcluster, "serial slave instance"=w2:refnum<class "Modbus Slave.lvclass">)  [unwired: 5 in]
  n144 = call-poly <vilib>:"Create Modbus Instance.vi"("serial type"=enum16{"RTU", "ASCII"}."RTU", "parity (even)"=w39, "unit ID"=w53, "baud rate (9600)"=w40, "VISA resource name"=w41) -> ("error out"=w51:errorcluster, "serial slave instance"=w52:refnum<class "Modbus Slave.lvclass">)  [unwired: 5 in]
  n145 = call-poly <vilib>:"Create Modbus Instance.vi"("serial type"=enum16{"RTU", "ASCII"}."RTU", "parity (even)"=w44, "unit ID"=w47, "baud rate (9600)"=w48, "VISA resource name"=w49) -> ("error out"=w45:errorcluster, "serial slave instance"=w46:refnum<class "Modbus Slave.lvclass">)  [unwired: 5 in]
  n146 = while "While循环" {
    shift-right: [w434] -> w19
    shift-left: w22 -> [w437]
    shift-right: [w431] -> w20
    shift-left: w21 -> [w436]
    shift-right: [w424] -> w86
    shift-left: w88 -> [w428]
    shift-right: [w423] -> w85
    shift-left: w87 -> [w427]
    stop <- FALSE stop-if-true
    # "R0步骤"
    # "300 1启动0空闲2停止"
    # "寄存器"
    # "100~20参数"
    # "M"
    # "X"
    # "Y"
    # "2500~2516输入线圈"
    # "100~116输入线圈"
    # "线圈"
    # "寄存器"
    # "0~32输出线圈"
    # "3840~3846模拟量"
    # "0~32运行状态"
    # "写"
    # "读"
    # "采配水与上位机通讯"
    n147 = Dequeue Element(queue=w428, error in (no error)=w427) -> (queue out=w426:refnum<queue>, element=w422:T2, error out=w425:errorcluster)  [unwired: 1 in, 1 out]
    n148 = case shown="\"串口重开\"" "采配水串口重开" {
      tunnel: w437 -> [w446 _]
      tunnel: w436 -> [w445 w534]
      tunnel: [w444 w520] -> w434
      tunnel: [w443 w521] -> w431
      tunnel: w426 -> [w441 w531]
      tunnel: w425 -> [w440 w530]
      tunnel: [w439 w529] -> w424
      tunnel: [w438 w528] -> w423
      tunnel: w422 -> [w442 _]
      frame "不重开", Default {
        n149 = case shown="\"write register\", 默认" w442 {
          tunnel: w446 -> [w460 w466 w489 w493 w516]
          tunnel: w445 -> [w459 w465 w488 w492 w515]
          tunnel: [w448 w464 w481 w491 w514] -> w444
          tunnel: [w447 w463 w480 w490 w513] -> w443
          tunnel: w441 -> [w458 w470 w478 w507 w512]
          tunnel: w440 -> [w457 w469 w477 w506 w511]
          tunnel: [w456 w468 w476 w505 w510] -> w439
          tunnel: [w455 w467 w475 w504 w509] -> w438
          frame "write register", Default {
            n150 = call-dynamic "Write Multiple Holding Registers.vi"("error in"=w459, "registers to write"=u16[] [0] ("holding register values"), "starting address"=u16 300, "Modbus slave in"=w460) -> ("error out"=w449:errorcluster, "Modbus slave out"=w450:refnum<class "Modbus Slave.lvclass">)  [unwired: 6 in]
            n151 = global read "采配水全局.vi" "参数设置"() -> (w452:T10)
            n152 = Cluster To Array(cluster=w452) -> (array=w451:i16[])
            n153 = call-dynamic "Write Multiple Holding Registers.vi"("error in"=w449, "registers to write"=w451, "starting address"=u16 100 ("read count"), "Modbus slave in"=w450) -> ("error out"=w447:errorcluster, "Modbus slave out"=w448:refnum<class "Modbus Slave.lvclass">)  [unwired: 6 in]
            n154 = Enqueue Element(queue=w458, element=T2."write and read register", error in (no error)=w457) -> (queue out=w456:refnum<queue>, error out=w455:errorcluster)  [unwired: 1 in, 1 out]
          }
          frame "read register" {
            n155 = call-dynamic "Read Holding Registers.vi"("error in"=w465, "number of inputs"=u16 4 ("number of holding registers"), "starting address"=u16 100, "Modbus slave in"=w466) -> ("error out"=w463:errorcluster, "Modbus slave out"=w464:refnum<class "Modbus Slave.lvclass">)  [unwired: 5 in, 1 out]
            n156 = Enqueue Element(queue=w470, element=T2."write and read register", error in (no error)=w469) -> (queue out=w468:refnum<queue>, error out=w467:errorcluster)  [unwired: 1 in, 1 out]
          }
          frame "write and read register" {
            n157 = global read "采配水全局.vi" "状态"() -> (w485:T11)
            n158 = Cluster To Array(cluster=w485) -> (array=w484:i16[])
            n159 = call-dynamic "Write and Read Multiple Holding Registers.vi"("read count"=u16 1, "read starting address"=u16 300 ("read count"), "error in"=w488, "write values"=w484, "write starting address"=u16 0 ("write operation starting address"), "Modbus instance in"=w489) -> ("error out"=w480:errorcluster, "read values"=w482:u16[], "Modbus instance out"=w481:refnum<class "Modbus Slave.lvclass">)  [unwired: 3 in]
            n160 = Index Array(array=w482) -> (element=w474:u16)  [unwired: 1 in]
            n161 = Enqueue Element(queue=w478, element=T2."write and read register", error in (no error)=w477) -> (queue out=w476:refnum<queue>, error out=w475:errorcluster)  [unwired: 1 in, 1 out]
            n162 = global write "采配水全局.vi" "启动模式"(w474) -> ()
          }
          frame "write coil" {
            n163 = global read "采配水全局.vi" "输出状态"() -> (w502:bool[])
            n164 = call-dynamic "Write Multiple Coils.vi"("error in"=w492, "coils to write"=w502, "starting address"=u16 0 ("write operation starting address"), "Modbus slave in"=w493) -> ("error out"=w500:errorcluster, "Modbus slave out"=w501:refnum<class "Modbus Slave.lvclass">)  [unwired: 6 in]
            n165 = global read "采配水全局.vi" "输入状态"() -> (w494:bool[])
            n166 = call-dynamic "Write Multiple Coils.vi"("error in"=w500, "coils to write"=w494, "starting address"=u16 100 ("read count"), "Modbus slave in"=w501) -> ("error out"=w498:errorcluster, "Modbus slave out"=w499:refnum<class "Modbus Slave.lvclass">)  [unwired: 6 in]
            n167 = Enqueue Element(queue=w507, element=T2."write and read register", error in (no error)=w506) -> (queue out=w505:refnum<queue>, error out=w504:errorcluster)  [unwired: 1 in, 1 out]
            n168 = global read "采配水全局.vi" "报警簇"() -> (w495:bool[])
            n169 = call-dynamic "Write Multiple Coils.vi"("error in"=w498, "coils to write"=w495, "starting address"=u16 2500 ("read count"), "Modbus slave in"=w499) -> ("error out"=w490:errorcluster, "Modbus slave out"=w491:refnum<class "Modbus Slave.lvclass">)  [unwired: 6 in]
          }
          frame "read coil" {
            n170 = call-dynamic "Read Coils.vi"("error in"=w515, "number of inputs"=u16 100 ("number of coils"), "starting address"=u16 0, "Modbus slave in"=w516) -> ("error out"=w513:errorcluster, "Modbus slave out"=w514:refnum<class "Modbus Slave.lvclass">)  [unwired: 5 in, 1 out]
            n171 = Enqueue Element(queue=w512, element=T2."write and read register", error in (no error)=w511) -> (queue out=w510:refnum<queue>, error out=w509:errorcluster)  [unwired: 1 in, 1 out]
          }
        }
      }
      frame "串口重开" {
        w526 = u16 0 items=["None", "Odd", "Even", "Mark", "Space"] ("parity (even)")
        n172 = call <vilib>:"Clear Errors.vi"("error in (no error)"=w534) -> ("error out"=w522:errorcluster)  [unwired: 5 in, 1 out]
        n173 = global read "采配水全局.vi" "采配水串口参数"() -> (w533:T1)
        n174 = Unbundle By Name(w533) -> ("VISA resource name"=w525:refnum<visa-resource-name>, "baud rate (设置)"=w524:u32, "unit ID"=w523:u8)
        n175 = Enqueue Element(queue=w531, element=T2."write and read register", error in (no error)=w530) -> (queue out=w529:refnum<queue>, error out=w528:errorcluster)  [unwired: 1 in, 1 out]
        n176 = call-poly <vilib>:"Create Modbus Instance.vi"("serial type"=enum16{"RTU", "ASCII"}."RTU", "parity (even)"=w526, "unit ID"=w523, "error in"=w522, "baud rate (9600)"=w524, "VISA resource name"=w525) -> ("error out"=w521:errorcluster, "serial slave instance"=w520:refnum<class "Modbus Slave.lvclass">)  [unwired: 4 in]
      }
    }
    n177 = Wait (ms)(milliseconds to wait=u32 1000 ("等待时间（毫秒）")) -> ()  [unwired: 1 out]
    n178 = Unbundle By Name(w431) -> ("status"=w430:bool)
    n179 = Not(x=w430) -> (.not. x?=→"采配水通讯":bool)
  }
  n180 = while "While循环" {
    shift-right: [w547] -> w38
    shift-left: w52 -> [w550]
    shift-right: [w543] -> w37
    shift-left: w51 -> [w549]
    shift-right: [w537] -> w66
    shift-left: w68 -> [w542]
    shift-right: [w536] -> w65
    shift-left: w67 -> [w541]
    stop <- FALSE stop-if-true
    # "1200H~12FFH控制命令区"
    # "读"
    # "写"
    # "10A0H~10E3H关键参数区"
    # "1080H~1090H状态告警区"
    # "1000H~1051H数据测量区"
    # "总氮与上位机通讯"
    n181 = Dequeue Element(queue=w542, error in (no error)=w541) -> (queue out=w539:refnum<queue>, element=w540:T2, error out=w538:errorcluster)  [unwired: 1 in, 1 out]
    n182 = Wait (ms)(milliseconds to wait=u32 1000 ("等待时间（毫秒）")) -> ()  [unwired: 1 out]
    n183 = case shown="\"串口重开\"" "总氮串口重开" {
      tunnel: w550 -> [w556 _]
      tunnel: w549 -> [w559 w645]
      tunnel: [w558 w635] -> w547
      tunnel: [w557 w633] -> w543
      tunnel: w540 -> [w555 _]
      tunnel: w539 -> [w554 w642]
      tunnel: w538 -> [w553 w641]
      tunnel: [w552 w640] -> w537
      tunnel: [w551 w639] -> w536
      frame "不重开", Default {
        n184 = case shown="\"write and read register\"" w555 {
          tunnel: w559 -> [w563 w573 w608 w616 w626]
          tunnel: [w562 w572 w597 w615 w625] -> w558
          tunnel: [w561 w571 w596 w614 w624] -> w557
          tunnel: w556 -> [w564 w574 w588 w617 w627]
          tunnel: w554 -> [w568 w580 w586 w612 w623]
          tunnel: w553 -> [w567 w579 w585 w611 w622]
          tunnel: [w566 w578 w584 w610 w621] -> w552
          tunnel: [w565 w577 w583 w609 w620] -> w551
          frame "write register", Default {
            n185 = call-dynamic "Write Multiple Holding Registers.vi"("error in"=w563, "registers to write"=u16[] [0] ("holding register values"), "starting address"=u16 4608 ("write operation starting address"), "Modbus slave in"=w564) -> ("error out"=w561:errorcluster, "Modbus slave out"=w562:refnum<class "Modbus Slave.lvclass">)  [unwired: 6 in]
            n186 = Enqueue Element(queue=w568, element=T2."write and read register", error in (no error)=w567) -> (queue out=w566:refnum<queue>, error out=w565:errorcluster)  [unwired: 1 in, 1 out]
          }
          frame "read register" {
            n187 = call-dynamic "Read Holding Registers.vi"("error in"=w573, "number of inputs"=u16 4 ("number of holding registers"), "starting address"=u16 100, "Modbus slave in"=w574) -> ("error out"=w571:errorcluster, "Modbus slave out"=w572:refnum<class "Modbus Slave.lvclass">)  [unwired: 5 in, 1 out]
            n188 = Enqueue Element(queue=w580, element=T2."write and read register", error in (no error)=w579) -> (queue out=w578:refnum<queue>, error out=w577:errorcluster)  [unwired: 1 in, 1 out]
          }
          frame "write and read register" {
            n189 = global read "总氮全局.vi" "测量数据区输入"() -> (w591:T6)
            n190 = call "数据测量区转CDAB.vi"("测量数据区"=w591) -> ("输出数组"=w601:u16[])  [unwired: 10 in]
            n191 = call-dynamic "Write and Read Multiple Holding Registers.vi"("read count"=u16 1, "read starting address"=u16 4608 ("write operation starting address"), "error in"=w608, "write values"=w601, "write starting address"=u16 4096 ("write operation starting address"), "Modbus instance in"=w588) -> ("error out"=w603:errorcluster, "read values"=w593:u16[], "Modbus instance out"=w604:refnum<class "Modbus Slave.lvclass">)  [unwired: 3 in]
            n192 = call "WordToHex.vi"("WORD"=w593) -> ("数组"=w592:u16[])  [unwired: 10 in]
            n193 = global read "总氮全局.vi" "状态告警区输入"() -> (w590:T7)
            n194 = Enqueue Element(queue=w586, element=T2."write and read register", error in (no error)=w585) -> (queue out=w584:refnum<queue>, error out=w583:errorcluster)  [unwired: 1 in, 1 out]
            n195 = Index Array(array=w592) -> (element=w582:u16)  [unwired: 1 in]
            n196 = global write "总氮全局.vi" "启动模式"(w582) -> ()
            n197 = call "状态告警区转CDAB.vi"("状态告警区"=w590) -> ("输出数组"=w600:u16[])  [unwired: 10 in]
            n198 = global read "总氮全局.vi" "关键参数区输入"() -> (w589:T12)
            n199 = call-dynamic "Write Multiple Holding Registers.vi"("error in"=w603, "registers to write"=w600, "starting address"=u16 4224 ("write operation starting address"), "Modbus slave in"=w604) -> ("error out"=w598:errorcluster, "Modbus slave out"=w599:refnum<class "Modbus Slave.lvclass">)  [unwired: 6 in]
            n200 = call "关键参数区转CDAB.vi"("关键参数区"=w589) -> ("输出数组"=w595:u16[])  [unwired: 10 in]
            n201 = call-dynamic "Write Multiple Holding Registers.vi"("error in"=w598, "registers to write"=w595, "starting address"=u16 4256 ("write operation starting address"), "Modbus slave in"=w599) -> ("error out"=w596:errorcluster, "Modbus slave out"=w597:refnum<class "Modbus Slave.lvclass">)  [unwired: 6 in]
          }
          frame "write coil" {
            n202 = call-dynamic "Write Multiple Coils.vi"("error in"=w616, "coils to write"=bool[] [] ("coil values"), "starting address"=u16 0, "Modbus slave in"=w617) -> ("error out"=w614:errorcluster, "Modbus slave out"=w615:refnum<class "Modbus Slave.lvclass">)  [unwired: 6 in]
            n203 = Enqueue Element(queue=w612, element=T2."write and read register", error in (no error)=w611) -> (queue out=w610:refnum<queue>, error out=w609:errorcluster)  [unwired: 1 in, 1 out]
          }
          frame "read coil" {
            n204 = call-dynamic "Read Coils.vi"("error in"=w626, "number of inputs"=u16 100 ("number of coils"), "starting address"=u16 0, "Modbus slave in"=w627) -> ("error out"=w624:errorcluster, "Modbus slave out"=w625:refnum<class "Modbus Slave.lvclass">)  [unwired: 5 in, 1 out]
            n205 = Enqueue Element(queue=w623, element=T2."write and read register", error in (no error)=w622) -> (queue out=w621:refnum<queue>, error out=w620:errorcluster)  [unwired: 1 in, 1 out]
          }
        }
      }
      frame "串口重开" {
        w631 = u16 0 items=["无", "奇", "偶"] ("parity (Even)")
        n206 = call <vilib>:"Clear Errors.vi"("error in (no error)"=w645) -> ("error out"=w634:errorcluster)  [unwired: 5 in, 1 out]
        n207 = global read "总氮全局.vi" "总氮串口参数"() -> (w644:T1)
        n208 = Unbundle By Name(w644) -> ("VISA resource name"=w638:refnum<visa-resource-name>, "baud rate (设置)"=w632:u32, "unit ID"=w637:u8)
        n209 = Enqueue Element(queue=w642, element=T2."write and read register", error in (no error)=w641) -> (queue out=w640:refnum<queue>, error out=w639:errorcluster)  [unwired: 1 in, 1 out]
        n210 = call-poly <vilib>:"Create Modbus Instance.vi"("serial type"=enum16{"RTU", "ASCII"}."RTU", "parity (even)"=w631, "unit ID"=w637, "error in"=w634, "baud rate (9600)"=w632, "VISA resource name"=w638) -> ("error out"=w633:errorcluster, "serial slave instance"=w635:refnum<class "Modbus Slave.lvclass">)  [unwired: 4 in]
      }
    }
    n211 = Unbundle By Name(w543) -> ("status"=w544:bool)
    n212 = Not(x=w544) -> (.not. x?=→"总氮通讯":bool)
  }
  n213 = while "While循环" {
    shift-right: [w658] -> w43
    shift-left: w46 -> [w661]
    shift-right: [w654] -> w42
    shift-left: w45 -> [w660]
    shift-right: [w647] -> w56
    shift-left: w58 -> [w649]
    shift-right: [w646] -> w55
    shift-left: w57 -> [w648]
    stop <- FALSE stop-if-true
    # "1200H~12FFH控制命令区"
    # "读"
    # "写"
    # "10A0H~10E3H关键参数区"
    # "1080H~1090H状态告警区"
    # "1000H~1051H数据测量区"
    # "总磷与上位机通讯"
    n214 = Dequeue Element(queue=w649, error in (no error)=w648) -> (queue out=w651:refnum<queue>, element=w652:T2, error out=w650:errorcluster)  [unwired: 1 in, 1 out]
    n215 = Wait (ms)(milliseconds to wait=u32 1000 ("等待时间（毫秒）")) -> ()  [unwired: 1 out]
    n216 = case shown="\"串口重开\"" "总磷串口重开" {
      tunnel: w661 -> [w670 _]
      tunnel: w660 -> [w669 w756]
      tunnel: [w663 w754] -> w658
      tunnel: [w662 w753] -> w654
      tunnel: w652 -> [w668 _]
      tunnel: w651 -> [w667 w748]
      tunnel: w650 -> [w666 w747]
      tunnel: [w665 w746] -> w647
      tunnel: [w664 w745] -> w646
      frame "不重开", Default {
        n217 = case shown="\"write register\", 默认" w668 {
          tunnel: [w677 w687 w709 w728 w738] -> w663
          tunnel: [w676 w686 w708 w727 w737] -> w662
          tunnel: [w679 w691 w702 w725 w736] -> w665
          tunnel: [w678 w690 w701 w724 w735] -> w664
          tunnel: w670 -> [w674 w685 w696 w723 w734]
          tunnel: w669 -> [w673 w684 w695 w722 w733]
          tunnel: w667 -> [w672 w683 w694 w721 w732]
          tunnel: w666 -> [w671 w682 w693 w720 w731]
          frame "write register", Default {
            n218 = call-dynamic "Write Multiple Holding Registers.vi"("error in"=w673, "registers to write"=u16[] [0] ("holding register values"), "starting address"=u16 4608 ("write operation starting address"), "Modbus slave in"=w674) -> ("error out"=w676:errorcluster, "Modbus slave out"=w677:refnum<class "Modbus Slave.lvclass">)  [unwired: 6 in]
            n219 = Enqueue Element(queue=w672, element=T2."write and read register", error in (no error)=w671) -> (queue out=w679:refnum<queue>, error out=w678:errorcluster)  [unwired: 1 in, 1 out]
          }
          frame "read register" {
            n220 = call-dynamic "Read Holding Registers.vi"("error in"=w684, "number of inputs"=u16 4 ("number of holding registers"), "starting address"=u16 100, "Modbus slave in"=w685) -> ("error out"=w686:errorcluster, "Modbus slave out"=w687:refnum<class "Modbus Slave.lvclass">)  [unwired: 5 in, 1 out]
            n221 = Enqueue Element(queue=w683, element=T2."write and read register", error in (no error)=w682) -> (queue out=w691:refnum<queue>, error out=w690:errorcluster)  [unwired: 1 in, 1 out]
          }
          frame "write and read register" {
            n222 = global read "总磷全局.vi" "测量数据区输入"() -> (w699:T6)
            n223 = call "数据测量区转CDAB.vi"("测量数据区"=w699) -> ("输出数组"=w713:u16[])  [unwired: 10 in]
            n224 = call-dynamic "Write and Read Multiple Holding Registers.vi"("read count"=u16 1, "read starting address"=u16 4608 ("write operation starting address"), "error in"=w695, "write values"=w713, "write starting address"=u16 4096 ("write operation starting address"), "Modbus instance in"=w696) -> ("error out"=w715:errorcluster, "read values"=w705:u16[], "Modbus instance out"=w716:refnum<class "Modbus Slave.lvclass">)  [unwired: 3 in]
            n225 = call "WordToHex.vi"("WORD"=w705) -> ("数组"=w704:u16[])  [unwired: 10 in]
            n226 = Enqueue Element(queue=w694, element=T2."write and read register", error in (no error)=w693) -> (queue out=w702:refnum<queue>, error out=w701:errorcluster)  [unwired: 1 in, 1 out]
            n227 = global read "总磷全局.vi" "状态告警区输入"() -> (w698:T7)
            n228 = Index Array(array=w704) -> (element=w700:u16)  [unwired: 1 in]
            n229 = global write "总磷全局.vi" "启动模式"(w700) -> ()
            n230 = call "状态告警区转CDAB.vi"("状态告警区"=w698) -> ("输出数组"=w712:u16[])  [unwired: 10 in]
            n231 = call-dynamic "Write Multiple Holding Registers.vi"("error in"=w715, "registers to write"=w712, "starting address"=u16 4224 ("write operation starting address"), "Modbus slave in"=w716) -> ("error out"=w710:errorcluster, "Modbus slave out"=w711:refnum<class "Modbus Slave.lvclass">)  [unwired: 6 in]
            n232 = global read "总磷全局.vi" "关键参数区输入"() -> (w697:T12)
            n233 = call "关键参数区转CDAB.vi"("关键参数区"=w697) -> ("输出数组"=w707:u16[])  [unwired: 10 in]
            n234 = call-dynamic "Write Multiple Holding Registers.vi"("error in"=w710, "registers to write"=w707, "starting address"=u16 4256 ("write operation starting address"), "Modbus slave in"=w711) -> ("error out"=w708:errorcluster, "Modbus slave out"=w709:refnum<class "Modbus Slave.lvclass">)  [unwired: 6 in]
          }
          frame "write coil" {
            n235 = call-dynamic "Write Multiple Coils.vi"("error in"=w722, "coils to write"=bool[] [] ("coil values"), "starting address"=u16 0, "Modbus slave in"=w723) -> ("error out"=w727:errorcluster, "Modbus slave out"=w728:refnum<class "Modbus Slave.lvclass">)  [unwired: 6 in]
            n236 = Enqueue Element(queue=w721, element=T2."write and read register", error in (no error)=w720) -> (queue out=w725:refnum<queue>, error out=w724:errorcluster)  [unwired: 1 in, 1 out]
          }
          frame "read coil" {
            n237 = call-dynamic "Read Coils.vi"("error in"=w733, "number of inputs"=u16 100 ("number of coils"), "starting address"=u16 0, "Modbus slave in"=w734) -> ("error out"=w737:errorcluster, "Modbus slave out"=w738:refnum<class "Modbus Slave.lvclass">)  [unwired: 5 in, 1 out]
            n238 = Enqueue Element(queue=w732, element=T2."write and read register", error in (no error)=w731) -> (queue out=w736:refnum<queue>, error out=w735:errorcluster)  [unwired: 1 in, 1 out]
          }
        }
      }
      frame "串口重开" {
        w742 = u16 0 items=["无", "奇", "偶"] ("parity (Even)")
        n239 = call <vilib>:"Clear Errors.vi"("error in (no error)"=w756) -> ("error out"=w755:errorcluster)  [unwired: 5 in, 1 out]
        n240 = global read "总磷全局.vi" "总磷串口参数"() -> (w750:T1)
        n241 = Unbundle By Name(w750) -> ("VISA resource name"=w744:refnum<visa-resource-name>, "baud rate (设置)"=w743:u32, "unit ID"=w752:u8)
        n242 = call-poly <vilib>:"Create Modbus Instance.vi"("serial type"=enum16{"RTU", "ASCII"}."RTU", "parity (even)"=w742, "unit ID"=w752, "error in"=w755, "baud rate (9600)"=w743, "VISA resource name"=w744) -> ("error out"=w753:errorcluster, "serial slave instance"=w754:refnum<class "Modbus Slave.lvclass">)  [unwired: 4 in]
        n243 = Enqueue Element(queue=w748, element=T2."write and read register", error in (no error)=w747) -> (queue out=w746:refnum<queue>, error out=w745:errorcluster)  [unwired: 1 in, 1 out]
      }
    }
    n244 = Unbundle By Name(w654) -> ("status"=w655:bool)
    n245 = Not(x=w655) -> (.not. x?=→"总磷通讯":bool)
  }
  n246 = while "While循环" {
    shift-right: [w769] -> w29
    shift-left: w31 -> [w772]
    shift-right: [w766] -> w28
    shift-left: w30 -> [w771]
    shift-right: [w759] -> w76
    shift-left: w78 -> [w764]
    shift-right: [w758] -> w75
    shift-left: w77 -> [w763]
    stop <- FALSE stop-if-true
    # "1200H~12FFH控制命令区"
    # "读"
    # "写"
    # "10A0H~10E3H关键参数区"
    # "1080H~1090H状态告警区"
    # "1000H~1051H数据测量区"
    # "氨氮与上位机通讯"
    n247 = Dequeue Element(queue=w764, error in (no error)=w763) -> (queue out=w761:refnum<queue>, element=w762:T2, error out=w760:errorcluster)  [unwired: 1 in, 1 out]
    n248 = case shown="\"串口重开\"" "氨氮串口重开" {
      tunnel: w772 -> [w781 _]
      tunnel: w771 -> [w780 w867]
      tunnel: [w779 w856] -> w769
      tunnel: [w778 w855] -> w766
      tunnel: w762 -> [w777 _]
      tunnel: w761 -> [w776 w864]
      tunnel: w760 -> [w775 w863]
      tunnel: [w774 w862] -> w759
      tunnel: [w773 w861] -> w758
      frame "不重开", Default {
        n249 = case shown="\"write and read register\"" w777 {
          tunnel: w781 -> [w789 w800 w830 w834 w849]
          tunnel: w780 -> [w788 w799 w829 w833 w848]
          tunnel: [w787 w794 w818 w832 w847] -> w779
          tunnel: [w786 w793 w817 w831 w846] -> w778
          tunnel: w776 -> [w785 w798 w808 w840 w845]
          tunnel: w775 -> [w784 w797 w807 w839 w844]
          tunnel: [w783 w796 w806 w838 w843] -> w774
          tunnel: [w782 w795 w805 w837 w842] -> w773
          frame "write register", Default {
            n250 = call-dynamic "Write Multiple Holding Registers.vi"("error in"=w788, "registers to write"=u16[] [0] ("holding register values"), "starting address"=u16 4608 ("write operation starting address"), "Modbus slave in"=w789) -> ("error out"=w786:errorcluster, "Modbus slave out"=w787:refnum<class "Modbus Slave.lvclass">)  [unwired: 6 in]
            n251 = Enqueue Element(queue=w785, element=T2."write and read register", error in (no error)=w784) -> (queue out=w783:refnum<queue>, error out=w782:errorcluster)  [unwired: 1 in, 1 out]
          }
          frame "read register" {
            n252 = call-dynamic "Read Holding Registers.vi"("error in"=w799, "number of inputs"=u16 4 ("number of holding registers"), "starting address"=u16 100, "Modbus slave in"=w800) -> ("error out"=w793:errorcluster, "Modbus slave out"=w794:refnum<class "Modbus Slave.lvclass">)  [unwired: 5 in, 1 out]
            n253 = Enqueue Element(queue=w798, element=T2."write and read register", error in (no error)=w797) -> (queue out=w796:refnum<queue>, error out=w795:errorcluster)  [unwired: 1 in, 1 out]
          }
          frame "write and read register" {
            n254 = global read "氨氮全局.vi" "测量数据区输入"() -> (w814:T6)
            n255 = call "数据测量区转CDAB.vi"("测量数据区"=w814) -> ("输出数组"=w822:u16[])  [unwired: 10 in]
            n256 = call-dynamic "Write and Read Multiple Holding Registers.vi"("read count"=u16 1, "read starting address"=u16 4608 ("write operation starting address"), "error in"=w829, "write values"=w822, "write starting address"=u16 4096 ("write operation starting address"), "Modbus instance in"=w830) -> ("error out"=w824:errorcluster, "read values"=w811:u16[], "Modbus instance out"=w825:refnum<class "Modbus Slave.lvclass">)  [unwired: 3 in]
            n257 = call "WordToHex.vi"("WORD"=w811) -> ("数组"=w810:u16[])  [unwired: 10 in]
            n258 = global read "氨氮全局.vi" "状态告警区输入"() -> (w813:T7)
            n259 = Index Array(array=w810) -> (element=w804:u16)  [unwired: 1 in]
            n260 = Enqueue Element(queue=w808, element=T2."write and read register", error in (no error)=w807) -> (queue out=w806:refnum<queue>, error out=w805:errorcluster)  [unwired: 1 in, 1 out]
            n261 = global write "氨氮全局.vi" "启动模式"(w804) -> ()
            n262 = call "状态告警区转CDAB.vi"("状态告警区"=w813) -> ("输出数组"=w821:u16[])  [unwired: 10 in]
            n263 = call-dynamic "Write Multiple Holding Registers.vi"("error in"=w824, "registers to write"=w821, "starting address"=u16 4224 ("write operation starting address"), "Modbus slave in"=w825) -> ("error out"=w819:errorcluster, "Modbus slave out"=w820:refnum<class "Modbus Slave.lvclass">)  [unwired: 6 in]
            n264 = global read "氨氮全局.vi" "关键参数区输入"() -> (w812:T12)
            n265 = call "关键参数区转CDAB.vi"("关键参数区"=w812) -> ("输出数组"=w816:u16[])  [unwired: 10 in]
            n266 = call-dynamic "Write Multiple Holding Registers.vi"("error in"=w819, "registers to write"=w816, "starting address"=u16 4256 ("write operation starting address"), "Modbus slave in"=w820) -> ("error out"=w817:errorcluster, "Modbus slave out"=w818:refnum<class "Modbus Slave.lvclass">)  [unwired: 6 in]
          }
          frame "write coil" {
            n267 = Enqueue Element(queue=w840, element=T2."write and read register", error in (no error)=w839) -> (queue out=w838:refnum<queue>, error out=w837:errorcluster)  [unwired: 1 in, 1 out]
            n268 = call-dynamic "Write Multiple Coils.vi"("error in"=w833, "coils to write"=bool[] [] ("coil values"), "starting address"=u16 0, "Modbus slave in"=w834) -> ("error out"=w831:errorcluster, "Modbus slave out"=w832:refnum<class "Modbus Slave.lvclass">)  [unwired: 6 in]
          }
          frame "read coil" {
            n269 = call-dynamic "Read Coils.vi"("error in"=w848, "number of inputs"=u16 100 ("number of coils"), "starting address"=u16 0, "Modbus slave in"=w849) -> ("error out"=w846:errorcluster, "Modbus slave out"=w847:refnum<class "Modbus Slave.lvclass">)  [unwired: 5 in, 1 out]
            n270 = Enqueue Element(queue=w845, element=T2."write and read register", error in (no error)=w844) -> (queue out=w843:refnum<queue>, error out=w842:errorcluster)  [unwired: 1 in, 1 out]
          }
        }
      }
      frame "串口重开" {
        w859 = u16 0 items=["None", "Odd", "Even", "Mark", "Space"] ("parity (even)")
        n271 = call <vilib>:"Clear Errors.vi"("error in (no error)"=w867) -> ("error out"=w857:errorcluster)  [unwired: 5 in, 1 out]
        n272 = global read "氨氮全局.vi" "氨氮串口参数"() -> (w866:T1)
        n273 = Unbundle By Name(w866) -> ("VISA resource name"=w858:refnum<visa-resource-name>, "baud rate (设置)"=w854:u32, "unit ID"=w853:u8)
        n274 = Enqueue Element(queue=w864, element=T2."write and read register", error in (no error)=w863) -> (queue out=w862:refnum<queue>, error out=w861:errorcluster)  [unwired: 1 in, 1 out]
        n275 = call-poly <vilib>:"Create Modbus Instance.vi"("serial type"=enum16{"RTU", "ASCII"}."RTU", "parity (even)"=w859, "unit ID"=w853, "error in"=w857, "baud rate (9600)"=w854, "VISA resource name"=w858) -> ("error out"=w855:errorcluster, "serial slave instance"=w856:refnum<class "Modbus Slave.lvclass">)  [unwired: 4 in]
      }
    }
    n276 = Wait (ms)(milliseconds to wait=u32 1000 ("等待时间（毫秒）")) -> ()  [unwired: 1 out]
    n277 = Unbundle By Name(w766) -> ("status"=w765:bool)
    n278 = Not(x=w765) -> (.not. x?=→"氨氮通讯":bool)
  }
  n279 = while "While循环" {
    shift-right: [w882] -> w8
    shift-left: w2 -> [w885]
    shift-right: [w878] -> w9
    shift-left: w1 -> [w884]
    shift-right: [w873] -> w97
    shift-left: w106 -> [w871]
    shift-right: [w872] -> w96
    shift-left: w105 -> [w870]
    stop <- FALSE stop-if-true
    # "1200H~12FFH控制命令区"
    # "读"
    # "写"
    # "10A0H~10E3H关键参数区"
    # "1080H~1090H状态告警区"
    # "1000H~1051H数据测量区"
    # "CODCr与上位机通讯"
    n280 = Get Queue Status(queue=w871, error in (no error)=w870) -> (queue out=w868:refnum<queue>, error out=w869:errorcluster)  [unwired: 1 in, 6 out]
    n281 = Dequeue Element(queue=w868, error in (no error)=w869) -> (queue out=w875:refnum<queue>, element=w876:T2, error out=w874:errorcluster)  [unwired: 1 in, 1 out]
    n282 = Wait (ms)(milliseconds to wait=u32 1000 ("等待时间（毫秒）")) -> ()  [unwired: 1 out]
    n283 = case shown="\"串口重开\"" "CODCr串口重开" {
      tunnel: w885 -> [w891 _]
      tunnel: w884 -> [w894 w979]
      tunnel: [w893 w966] -> w882
      tunnel: [w892 w967] -> w878
      tunnel: w876 -> [w890 _]
      tunnel: w875 -> [w889 w976]
      tunnel: w874 -> [w888 w975]
      tunnel: [w887 w974] -> w873
      tunnel: [w886 w973] -> w872
      frame "不重开", Default {
        n284 = case shown="\"write and read register\"" w890 {
          tunnel: w894 -> [w902 w908 w942 w949 w956]
          tunnel: [w901 w907 w931 w948 w955] -> w893
          tunnel: [w900 w906 w930 w947 w954] -> w892
          tunnel: w891 -> [w903 w909 w927 w950 w957]
          tunnel: w889 -> [w899 w913 w922 w946 w961]
          tunnel: w888 -> [w898 w912 w921 w945 w960]
          tunnel: [w897 w911 w920 w944 w959] -> w887
          tunnel: [w896 w910 w919 w943 w958] -> w886
          frame "write register", Default {
            n285 = call-dynamic "Write Multiple Holding Registers.vi"("error in"=w902, "registers to write"=u16[] [0] ("holding register values"), "starting address"=u16 4608 ("write operation starting address"), "Modbus slave in"=w903) -> ("error out"=w900:errorcluster, "Modbus slave out"=w901:refnum<class "Modbus Slave.lvclass">)  [unwired: 6 in]
            n286 = Enqueue Element(queue=w899, element=T2."write and read register", error in (no error)=w898) -> (queue out=w897:refnum<queue>, error out=w896:errorcluster)  [unwired: 1 in, 1 out]
          }
          frame "read register" {
            n287 = call-dynamic "Read Holding Registers.vi"("error in"=w908, "number of inputs"=u16 4 ("number of holding registers"), "starting address"=u16 100, "Modbus slave in"=w909) -> ("error out"=w906:errorcluster, "Modbus slave out"=w907:refnum<class "Modbus Slave.lvclass">)  [unwired: 5 in, 1 out]
            n288 = Enqueue Element(queue=w913, element=T2."write and read register", error in (no error)=w912) -> (queue out=w911:refnum<queue>, error out=w910:errorcluster)  [unwired: 1 in, 1 out]
          }
          frame "write and read register" {
            n289 = global read "CODCr全局.vi" "测量数据区输入"() -> (w926:T6)
            n290 = call "数据测量区转CDAB.vi"("测量数据区"=w926) -> ("输出数组"=w935:u16[])  [unwired: 10 in]
            n291 = call-dynamic "Write and Read Multiple Holding Registers.vi"("read count"=u16 1, "read starting address"=u16 4608 ("write operation starting address"), "error in"=w942, "write values"=w935, "write starting address"=u16 4096 ("write operation starting address"), "Modbus instance in"=w927) -> ("error out"=w937:errorcluster, "read values"=w918:u16[], "Modbus instance out"=w938:refnum<class "Modbus Slave.lvclass">)  [unwired: 3 in]
            n292 = global read "CODCr全局.vi" "状态告警区输入"() -> (w925:T7)
            n293 = Index Array(array=w918) -> (element=w917:u16)  [unwired: 1 in]
            n294 = Enqueue Element(queue=w922, element=T2."write and read register", error in (no error)=w921) -> (queue out=w920:refnum<queue>, error out=w919:errorcluster)  [unwired: 1 in, 1 out]
            n295 = call "状态告警区转CDAB.vi"("状态告警区"=w925) -> ("输出数组"=w934:u16[])  [unwired: 10 in]
            n296 = global read "CODCr全局.vi" "关键参数区输入"() -> (w924:T12)
            n297 = call-dynamic "Write Multiple Holding Registers.vi"("error in"=w937, "registers to write"=w934, "starting address"=u16 4224 ("write operation starting address"), "Modbus slave in"=w938) -> ("error out"=w932:errorcluster, "Modbus slave out"=w933:refnum<class "Modbus Slave.lvclass">)  [unwired: 6 in]
            n298 = call "关键参数区转CDAB.vi"("关键参数区"=w924) -> ("输出数组"=w929:u16[])  [unwired: 10 in]
            n299 = global write "CODCr全局.vi" "启动模式"(w917) -> ()
            n300 = call-dynamic "Write Multiple Holding Registers.vi"("error in"=w932, "registers to write"=w929, "starting address"=u16 4256 ("write operation starting address"), "Modbus slave in"=w933) -> ("error out"=w930:errorcluster, "Modbus slave out"=w931:refnum<class "Modbus Slave.lvclass">)  [unwired: 6 in]
          }
          frame "write coil" {
            n301 = call-dynamic "Write Multiple Coils.vi"("error in"=w949, "coils to write"=bool[] [] ("coil values"), "starting address"=u16 0, "Modbus slave in"=w950) -> ("error out"=w947:errorcluster, "Modbus slave out"=w948:refnum<class "Modbus Slave.lvclass">)  [unwired: 6 in]
            n302 = Enqueue Element(queue=w946, element=T2."write and read register", error in (no error)=w945) -> (queue out=w944:refnum<queue>, error out=w943:errorcluster)  [unwired: 1 in, 1 out]
          }
          frame "read coil" {
            n303 = call-dynamic "Read Coils.vi"("error in"=w956, "number of inputs"=u16 100 ("number of coils"), "starting address"=u16 0, "Modbus slave in"=w957) -> ("error out"=w954:errorcluster, "Modbus slave out"=w955:refnum<class "Modbus Slave.lvclass">)  [unwired: 5 in, 1 out]
            n304 = Enqueue Element(queue=w961, element=T2."write and read register", error in (no error)=w960) -> (queue out=w959:refnum<queue>, error out=w958:errorcluster)  [unwired: 1 in, 1 out]
          }
        }
      }
      frame "串口重开" {
        w971 = u16 0 items=["None", "Odd", "Even", "Mark", "Space"] ("parity (even)")
        n305 = call <vilib>:"Clear Errors.vi"("error in (no error)"=w979) -> ("error out"=w968:errorcluster)  [unwired: 5 in, 1 out]
        n306 = global read "CODCr全局.vi" "CODCr串口参数"() -> (w978:T1)
        n307 = Unbundle By Name(w978) -> ("VISA resource name"=w970:refnum<visa-resource-name>, "baud rate (设置)"=w969:u32, "unit ID"=w965:u8)
        n308 = Enqueue Element(queue=w976, element=T2."write and read register", error in (no error)=w975) -> (queue out=w974:refnum<queue>, error out=w973:errorcluster)  [unwired: 1 in, 1 out]
        n309 = call-poly <vilib>:"Create Modbus Instance.vi"("serial type"=enum16{"RTU", "ASCII"}."RTU", "parity (even)"=w971, "unit ID"=w965, "error in"=w968, "baud rate (9600)"=w969, "VISA resource name"=w970) -> ("error out"=w967:errorcluster, "serial slave instance"=w966:refnum<class "Modbus Slave.lvclass">)  [unwired: 4 in]
      }
    }
    n310 = Unbundle By Name(w878) -> ("status"=w879:bool)
    n311 = Not(x=w879) -> (.not. x?=→"CODCr通讯":bool)
  }
  n312 = while {
    tunnel: [w988] -> _
    tunnel: [w987] -> _
    tunnel: [w986] -> _
    stop <- FALSE stop-if-true
    # "1200H~12FFH控制命令区"
    # "读"
    # "写"
    # "100~103数据测量区"
    # "质控单元与上位机通讯"
    n313 = shared-variable "我的电脑\\OPC（MB）.lvlib\\质控1#R103"() -> (w980:u16, error out=w992:errorcluster)  [unwired: 1 in]
    n314 = shared-variable "我的电脑\\OPC（MB）.lvlib\\质控2#R103"() -> (w981:u16, error out=w994:errorcluster)  [unwired: 1 in]
    n315 = global read "质控单元全局.vi" "状态"() -> (w1000:T5)
    n316 = global read "质控单元2全局.vi" "状态"() -> (w1002:T5)
    n317 = Wait (ms)(milliseconds to wait=u32 1000 ("等待时间（毫秒）")) -> ()  [unwired: 1 out]
    n318 = Unbundle By Name(w1000) -> ("R0"=w1001:i16)
    n319 = Unbundle By Name(w1002) -> ("R0"=w1003:i16)
    n320 = Bundle By Name(cluster=cluster{"R0":i16} {"R0"=0} ("状态"), "R0"=w1001) -> (w999:cluster{"R0":i16})
    n321 = Bundle By Name(cluster=cluster{"R0":i16} {"R0"=0} ("状态"), "R0"=w1003) -> (w1005:cluster{"R0":i16})
    n322 = Cluster To Array(cluster=w1005) -> (array=w1006:i16[])
    n323 = Cluster To Array(cluster=w999) -> (array=w997:i16[])
    n324 = Index Array(array=w1006) -> (element=w1012:i16)  [unwired: 1 in]
    n325 = Index Array(array=w997) -> (element=w996:i16)  [unwired: 1 in]
    n326 = shared-variable "我的电脑\\OPC（MB）.lvlib\\质控2#R100"(w1012, error in=w994) -> (error out=w988:errorcluster)
    n327 = shared-variable "我的电脑\\OPC（MB）.lvlib\\质控1#R100"(w996, error in=w992) -> (error out=w986:errorcluster)
    n328 = global write "质控单元全局.vi" "启动模式"(w980) -> ()
    n329 = global write "质控单元2全局.vi" "启动模式"(w981) -> ()
    n330 = shared-variable "我的电脑\\OPC（MB）.lvlib\\质控3#R103"() -> (w982:u16, error out=w993:errorcluster)  [unwired: 1 in]
    n331 = global read "质控单元3全局.vi" "状态"() -> (w1011:T5)
    n332 = Unbundle By Name(w1011) -> ("R0"=w1010:i16)
    n333 = Bundle By Name(cluster=cluster{"R0":i16} {"R0"=0} ("状态"), "R0"=w1010) -> (w1008:cluster{"R0":i16})
    n334 = Cluster To Array(cluster=w1008) -> (array=w1007:i16[])
    n335 = Index Array(array=w1007) -> (element=w1013:i16)  [unwired: 1 in]
    n336 = shared-variable "我的电脑\\OPC（MB）.lvlib\\质控3#R100"(w1013, error in=w993) -> (error out=w987:errorcluster)
    n337 = global write "质控单元3全局.vi" "启动模式"(w982) -> ()
    n338 = Unbundle By Name(w986) -> ("status"=w990:bool)
    n339 = Unbundle By Name(w988) -> ("status"=w995:bool)
    n340 = Unbundle By Name(w987) -> ("status"=w991:bool)
    n341 = Not(x=w990) -> (.not. x?=w984:bool)
    n342 = Not(x=w995) -> (.not. x?=w989:bool)
    n343 = Not(x=w991) -> (.not. x?=w985:bool)
    n344 = Compound Arithmetic op=AND ("复合运算")(w989, w985, w984) -> (→"质控单元通讯":bool)
  }
  n345 = while {
    tunnel: w128 -> [w1020]
    tunnel: w127 -> [w1019]
    tunnel: [w1018] -> w126
    tunnel: [w1017] -> w125
    tunnel: w121 -> [w1016]
    stop <- FALSE stop-if-true
    n346 = event shown="[2] \"氨氮\", \"总氮\", \"总磷\", \"CODMn\", \"CODCr\", \"采配水\", \"质控单元\": 值改变" {
      selector: _ -> [_ _ _]
      dyn-events: _ -> [_ _ _]
      timeout: _ -> [_ _ _]
      tunnel: w1020 -> [w1023 _ _]
      tunnel: w1019 -> [w1022 _ _]
      tunnel: [w1023 _ _] -> w1018
      tunnel: [w1022 _ _] -> w1017
      tunnel: w1016 -> [_ _ w1027]
      event Timeout {
        n347 = event-data() -> ()  [unwired: 1 in, 3 out]
      }
      event "退出": Value Change {
        n348 = event-data() -> ()  [unwired: 1 in, 6 out]
        n349 = Stop(stop? (T)=TRUE ("停止？(T)")) -> ()
      }
      event "氨氮", "总氮", "总磷", "CODMn", "CODCr", "采配水", "质控单元": Value Change {
        n350 = event-data() -> ("CtlRef"=w1029:refnum<vi>)  [unwired: 1 in, 5 out]
        n351 = property class="Bool"(reference=w1029) -> ("BoolText.Text"=w1028:string)  [unwired: 1 in, 2 out]
        n352 = case shown="\"质控单元\"" w1028 {
          tunnel: [0 1 2 3 4 5 6] -> w1026
          frame "采配水", Default {
          }
          frame "氨氮" {
          }
          frame "总氮" {
          }
          frame "总磷" {
          }
          frame "CODMn" {
          }
          frame "CODCr" {
          }
          frame "质控单元" {
          }
        }
        n353 = Index Array(array=w1027, index=w1026) -> (element=w1025:refnum<vi>)
        n354 = invoke on="子面板" class="SubPnl" method="Remove VI"() -> (error out=w1030:errorcluster)  [unwired: 3 in, 2 out]
        n355 = invoke on="子面板" class="SubPnl" method="Insert VI"(error in=w1030, "VI Ref"=w1025) -> ()  [unwired: 2 in, 4 out]
      }
    }
  }
  n356 = Cancel Notification(0:w126, 3:w125) -> (8:w130:refnum<notifier>, 11:w129:errorcluster)  [unwired: 1 out]
  n357 = Release Notifier(notifier=w130, error in (no error)=w129) -> ()  [unwired: 1 in, 3 out]
  n358 = Release Queue(queue=w56, error in (no error)=w55) -> ()  [unwired: 1 in, 3 out]
  n359 = Release Queue(queue=w86, error in (no error)=w85) -> ()  [unwired: 1 in, 3 out]
  n360 = Release Queue(queue=w76, error in (no error)=w75) -> ()  [unwired: 1 in, 3 out]
  n361 = call-dynamic "Shutdown.vi"("error in"=w42, "Modbus slave in"=w43) -> ()  [unwired: 9 in, 1 out]
  n362 = Release Queue(queue=w95, error in (no error)=w94) -> ()  [unwired: 1 in, 3 out]
  n363 = call-dynamic "Shutdown.vi"("error in"=w10, "Modbus slave in"=w11) -> ()  [unwired: 9 in, 1 out]
  n364 = Release Queue(queue=w97, error in (no error)=w96) -> ()  [unwired: 1 in, 3 out]
  n365 = Release Queue(queue=w66, error in (no error)=w65) -> ()  [unwired: 1 in, 3 out]
  n366 = call-dynamic "Shutdown.vi"("error in"=w9, "Modbus slave in"=w8) -> ()  [unwired: 9 in, 1 out]
  n367 = call-dynamic "Shutdown.vi"("error in"=w20, "Modbus slave in"=w19) -> ()  [unwired: 9 in, 1 out]
  n368 = call-dynamic "Shutdown.vi"("error in"=w28, "Modbus slave in"=w29) -> ()  [unwired: 9 in, 1 out]
  n369 = call-dynamic "Shutdown.vi"("error in"=w37, "Modbus slave in"=w38) -> ()  [unwired: 9 in, 1 out]
